vi "GTcode_v6_simulISS_MAP.vi"() -> ()   [LabVIEW 2016]
uses:
  <vilib>/Utility/error.llb/DialogType.ctl
  <vilib>/Analysis/5stat.llb/RMS (DBL).vi
  <vilib>/Utility/config.llb/Write Key (String).vi
  <vilib>/Utility/config.llb/Write Key (U32).vi
  <vilib>/Utility/config.llb/Write Key (Double).vi
  <vilib>/Utility/config.llb/Write Key (I32).vi
  <vilib>/Utility/config.llb/Read Key (U32).vi
  <vilib>/Utility/config.llb/Read Key (I32).vi
  <vilib>/Waveform/WDTOps.llb/WDT Append Waveforms DBL.vi
  <vilib>/Utility/file.llb/Write Delimited Spreadsheet (string).vi
  <vilib>/Waveform/WDTFileIO.llb/Export Waveforms To Spreadsheet File (1D).vi
  <vilib>/Utility/config.llb/NI_LVConfig.lvlib
  <vilib>/Analysis/NI_AALPro.lvlib
panel:
  out "MARk Wvfm":waveform(dbl)(graph)
  out "ComboMaxArray":dbl[](array[numeric])
  out "Trial Data Column Headers":string[](array[string])
  in  "TrialDataRowHeaders":string[](array[string])=["Wfm1", "Wfm2", "Wfm3", "Wfm4", "Wfm5", "Wfm6", "Wfm7", "Wfm8"]
  out "SignalMaxArray":dbl[][](array[numeric])
  in  "CurrentMaxIndex":dbl
  out "SignalsAvgMaxArray":dbl[](array[numeric])
  in  "Mean%Index":dbl=4.0
  in  "%StdDevIndex":dbl=5.0
  in  "StdDevIndex":dbl=3.0
  in  "MeanIndex":dbl=2.0
  in  "MaxIndex":dbl=1.0
  in  "MinIndex":dbl
  out "Stability Data":dbl[][](array[numeric])
  out "trialFilteredData":waveform(dbl)[](array[waveform])
  out "filteredWaveforms":waveform(dbl)[](array[waveform])
  in  "ComboMaxAvg":dbl
  in  "End Program":bool
  out "Wfm1":waveform(dbl)(graph)
  out "Wfm2":waveform(dbl)(graph)
  out "Wfm3":waveform(dbl)(graph)
  out "Wfm4":waveform(dbl)(graph)
  out "Wfm5":waveform(dbl)(graph)
  out "Wfm6":waveform(dbl)(graph)
  out "Wfm7":waveform(dbl)(graph)
  out "Wfm8":waveform(dbl)(graph)
  out "RMS 1":dbl(graph)
  out "RMS 2":dbl(graph)
  out "RMS 3":dbl(graph)
  out "RMS 4":dbl(graph)
  out "RMS 5":dbl(graph)
  out "RMS 6":dbl(graph)
  out "RMS 7":dbl(graph)
  out "RMS 8":dbl(graph)
  out "CombinedMovingAvg":dbl
  out "LeftPercentActivation":dbl
  out "GetMaxStartTime":timestamp
  out "Aggregate1":waveform(dbl)[](array[waveform])
  out "Aggregate2":waveform(dbl)[](array[waveform])
  out "Aggregate3":waveform(dbl)[](array[waveform])
  out "Aggregate4":waveform(dbl)[](array[waveform])
  out "Aggregate5":waveform(dbl)[](array[waveform])
  out "Aggregate6":waveform(dbl)[](array[waveform])
  out "Aggregate7":waveform(dbl)[](array[waveform])
  out "Aggregate 8":waveform(dbl)[](array[waveform])
  in  "Tab Control":T1(tab)=enum."Real Time Fitting Parameters"
  in  "Fixed Time":bool
  in  "Detector Used":T2(ring)=enum."Det 2"
  in  "Real Time Fitting?":bool
  out "g2":cluster{"Delay Time":sgl[], sgl[]}[](graph) caption="Normalized Correlation Function"
  out "Tau":cluster{"tmp":dbl, dbl}(graph) caption="Relative Changes of Flow"
  in  "QUIT":bool
  in  "Clear plots":bool
  in  "Baseline":bool
  in  "MARK\nMark":bool
  in  "Stop":bool
  in  "Sequence Scan":bool
  out "Mark #":u32
  out "Trial #":u32
  out "Frame #":u32
  out "Det 8":sgl format="%.3f"
  out "Det 7":sgl format="%.3f"
  out "Det 6":sgl format="%.3f"
  out "Det 5":sgl format="%.3f"
  out "Det 4":sgl format="%.3f"
  out "Det 3":sgl format="%.3f"
  out "Det 2":sgl format="%.3f"
  out "Det 1":sgl format="%.3f"
  out "Computer Time":string="2010-1-12 23:16:10"
  in  "D1":bool
  in  "D2":bool
  in  "D3":bool
  in  "D4":bool
  in  "D5":bool
  in  "D6":bool
  in  "D7":bool
  in  "D8":bool
  in  "Fixed # of Frames":u32=5
  out "Status":string="Quit"
  in  "Optical Switch OPEN":bool
  in  "Delay between frames(ms)":u32=500
  out "Time Left (ms)":sgl format="%.3f"
  in  "Integration Time (ms)":sgl=1000.0 min=1 max=13000 step=1
  in  "File Name:":string="test0"
  in  "Data Save Directory:":path=path "C:/data"
  in  "ISS Lasers ON":bool
  in  "Test":bool
  out "DispLeftMovingAvg":dbl(slide) caption="EMG" max=1.0 scale=0.0..100.0
  in  "startGetMax":bool
  in  "resetMax":bool
  out "Trial In Progress":bool
  out "Acquiring Max":bool
  in  "Lines":tag="Dev1/port1/line0:1, Dev1/port1/line3:7"
  in  "Delaytime(ms)":u32=200
  in  "Initialize Correlator":bool
  in  "Detector Select":enum32{"4 Detectors", "8 Detectors"}(radio)=enum."8 Detectors"
  in  "Update Time (ms)\nDO NOT CHANGE!":u32=105 min=1 max=999 step=1
  in  "Laser Input Name":refnum<visa-resource-name>="COM7"
  in  "Visible Averages":bool[](array[boolean])=[FALSE, FALSE, FALSE, FALSE]
  in  "Avg":bool[][](array[boolean])=[[FALSE, FALSE, FALSE, FALSE, FALSE, FALSE, FALSE, FALSE], [FALSE, FALSE, FALSE, FALSE, FALSE, FALSE, FALSE, FALSE], [FALSE, FALSE, FALSE, FALSE, FALSE, FALSE, FALSE, FALSE], [FALSE, FALSE, FALSE, FALSE, FALSE, FALSE, FALSE, FALSE]]
  in  "Number Samples":dbl=50.0
  out "NIBP Data (*scaled by 98 to convert from V to mmHg)":dynamicdata(graph)
  in  "Record MAP data?":bool=TRUE
  in  "Sampling Rate (Hz)":dbl=100.0
  in  "ExternalADC":tag="Dev2"
  in  "Lower Cut-Off":dbl=20.0
  in  "Upper Cut-Off":dbl=300.0
  in  "Sample rate (Hz)":dbl=2000.0
  in  "Frames Per Second":dbl=30.0
  in  "Moving Average Length (s)":dbl=0.5
  in  "SignalB":dbl=2.0
  in  "SignalA":dbl=1.0
  in  "Target Percentage":dbl=10.0
  in  "Amplitude Error":dbl
  in  "NumberOfMaximumsInAverage":dbl=3.0
  in  "SecondsToAcquireMax":dbl=10.0
  in  "EMG Input Device\nProduct Type":string="USB-6009"
  out "raw data":dynamicdata(graph)
  out "Combined RMS":dbl(graph)
  out "Trial Raw Waveforms":waveform(dbl)[](graph)
  out "Bufffer Index":dbl
  out "Frames in Buffer":dbl
  out "Samples per frame":dbl
  out "Reset Data Acquisition\nAnd UI Updating":bool=TRUE
  in  "Extension":string="_EMG.txt"
  out "4CH?":bool
  out "Detector#":u32=1
  out "Source#":u32=1
  # "kHz"
  # "kHz"
  # "Maximums Data"
  # "Don't Change these Parameters unless you know clearly what you are doing"
  # "ISS Triggers Setup"
  # "Channel Parameters"
  # "Step1"
  # "Line"
  # "0"
  # "1"
  # "3"
  # "4"
  # "5"
  # "6"
  # "7"
  # "*The number of lines in the list must\nmatch the number of elements in\nthe array."
  # "Step2"
  # "Line"
  # "0"
  # "1"
  # "3"
  # "4"
  # "5"
  # "6"
  # "7"
  # "Step3"
  # "Line"
  # "0"
  # "1"
  # "3"
  # "4"
  # "5"
  # "6"
  # "7"
  # "Line    Signal\n\n0           ISS Trigger (0: OFF, 1: ON)\n1           Flow Laser 1 ON/OFF (0:OFF, 1:ON)\n2           ISS Data Acquisition (0: DONE, 1: NO)\n3           ISS Laser ON/OFF (0: ON, 1: OFF)\n4           Trigger for Marks  (0: OFF, 1: ON)\n5           Flow Laser 2 ON/OFF (0:OFF, 1:ON)\n6           Reserved\n7           Reserved"
  # "Wait ISS Data Acuisition DONE Signal"
  # "Step4"
  # "Step5"
  # "Line"
  # "0"
  # "1"
  # "3"
  # "4"
  # "5"
  # "6"
  # "7"
  # "Flow Lasers Setup"
  # "FROM FRONT PANEL"
  # "Line"
  # "0"
  # "1"
  # "3"
  # "4"
  # "5"
  # "6"
  # "7"
  # "Line"
  # "0"
  # "1"
  # "3"
  # "4"
  # "5"
  # "6"
  # "7"
  # "Det 1"
  # "Det 2"
  # "Det 3"
  # "Det 4"
  # "Det 5"
  # "Det 6"
  # "Det 7"
  # "Det 8"
  # "Avg 1"
  # "Avg 2"
  # "Avg 3"
  # "Avg 4"
  # "Db"
  # "Beta"
  # "Mua"
  # "MuS'"
  # "1"
  # "2"
  # "3"
  # "4"
  # "5"
  # "6"
  # "7"
  # "8"
  # "Avg 1"
  # "Starting Pt"
  # "End Pt"
  # "Approximate"
  # "Variables"
  # "Avg 2"
  # "Avg 3"
  # "Avg 4"
  # "Source Detector  Separations"
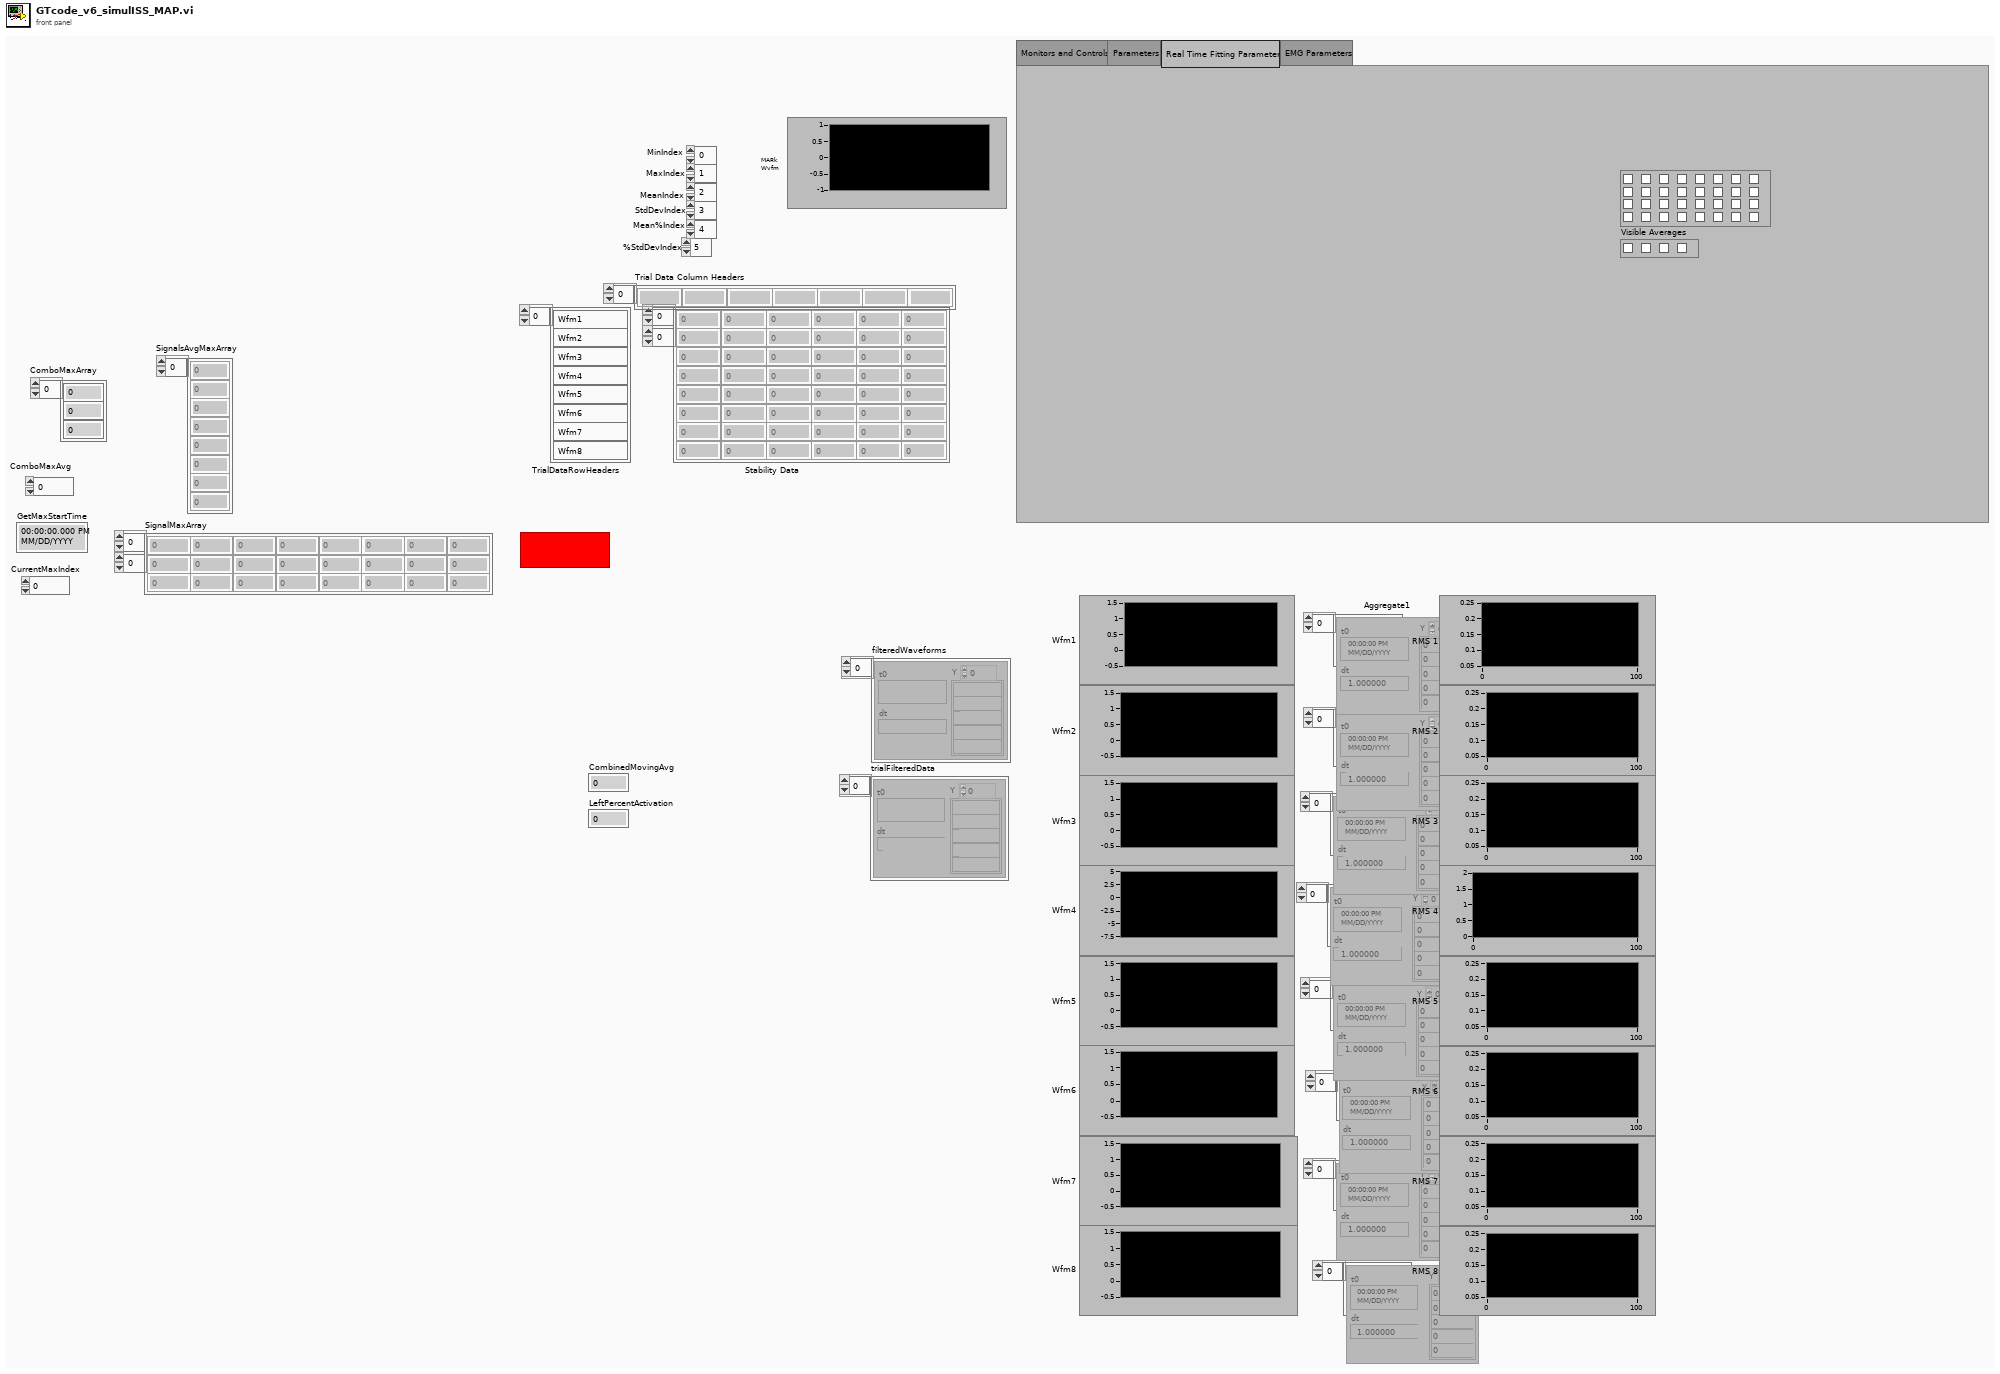
[diagram p1: front panel]
types:
  T1 = enum32{"Monitors and Controls", "Parameters", "Real Time Fitting Parameters", "EMG Parameters"}
  T2 = enum16{"Det 1", "Det 2", "Det 3", "Det 4", "Det 5", "Det 6", "Det 7", "Det 8"}
  T3 = typedef "DialogType.ctl" = u16
  T4 = typedef "WaveformArrayControl.ctl" = waveform(dbl)[]
  T5 = enum8{"Enabled", "Disabled", "Disabled and Grayed Out"}
  T6 = cluster{dbl, dbl, dbl, dbl, dbl, dbl, dbl, dbl, dbl, dbl, dbl, dbl}
  T7 = typedef "NI_LVConfig.lvlib/Config Data RefNum.ctl" = refnum<k1>
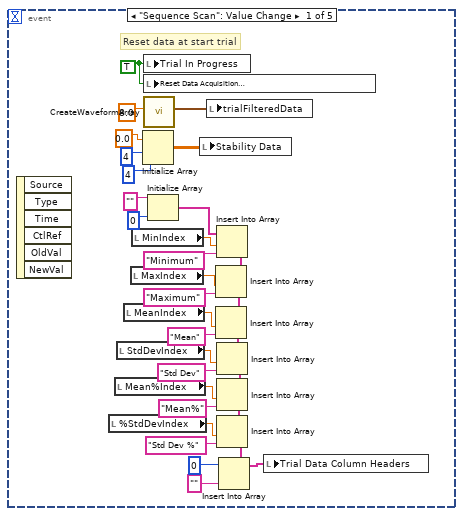
[diagram p2: hidden frame]
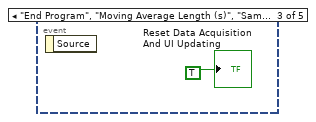
[diagram p5: hidden frame]
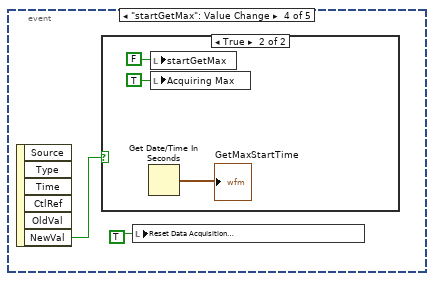
[diagram p6: hidden frame]
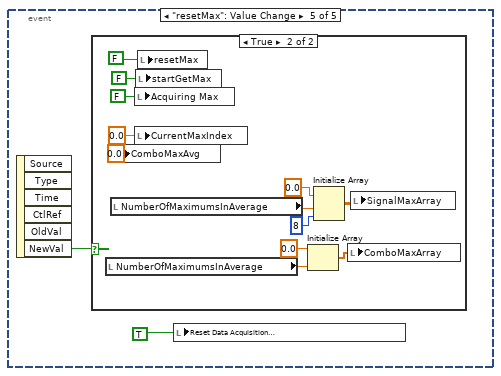
[diagram p8: hidden frame]
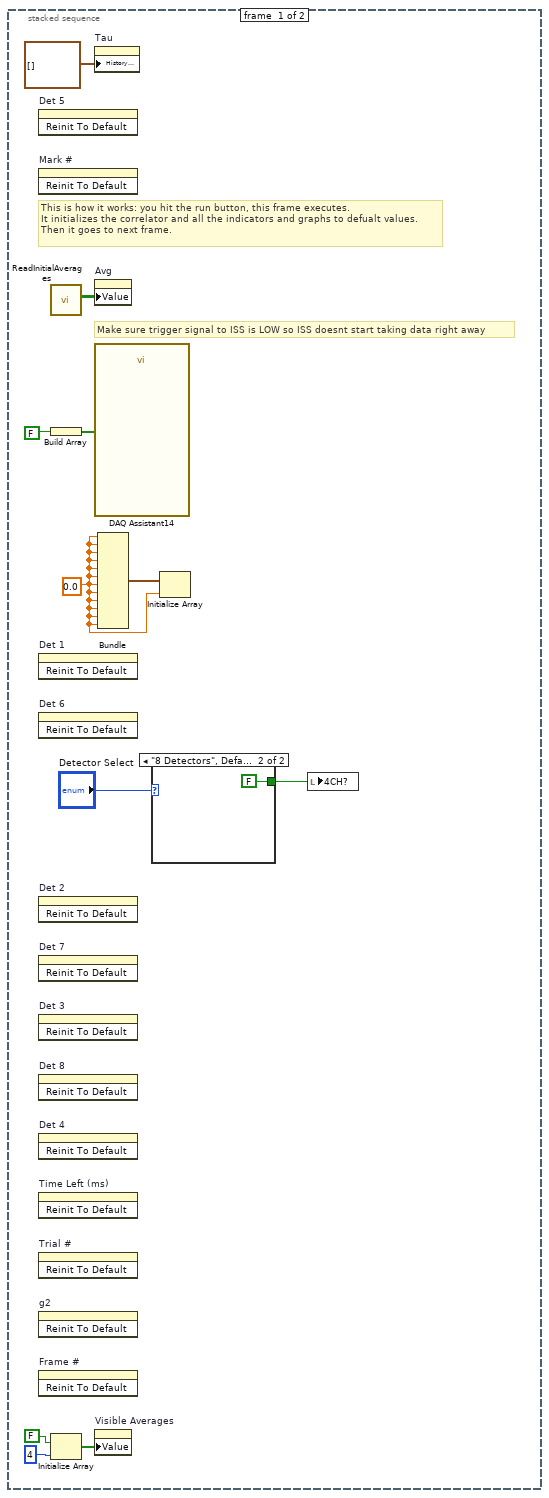
[diagram p15: hidden frame]
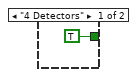
[diagram p16: hidden frame]
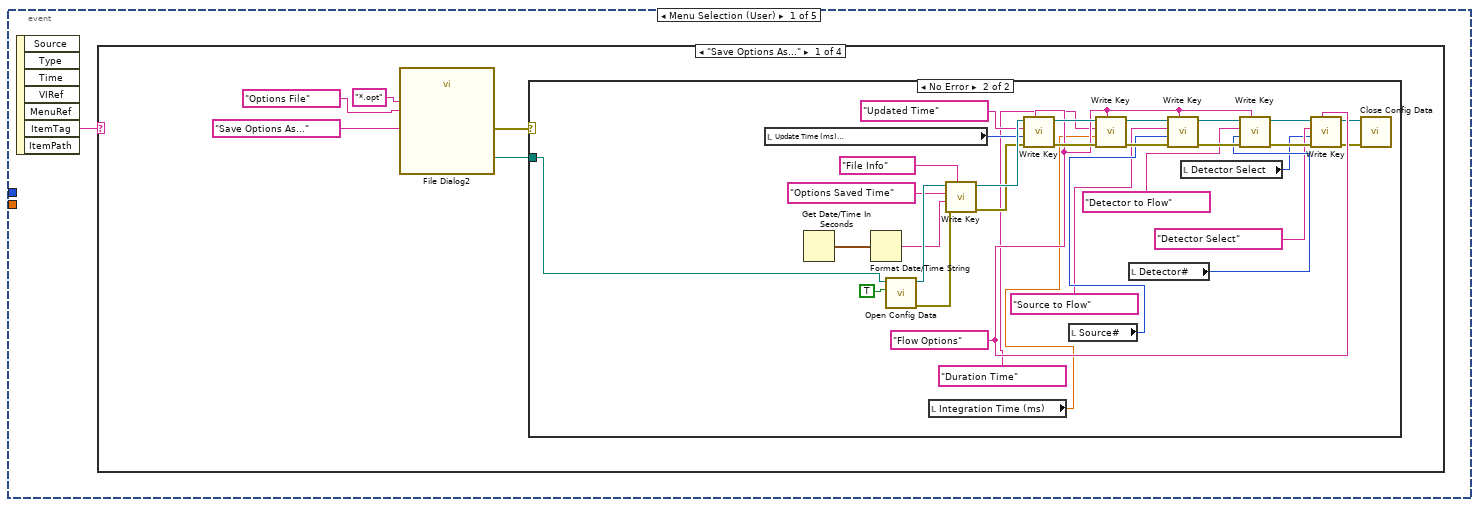
[diagram p17: hidden frame]
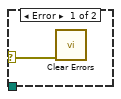
[diagram p18: hidden frame]
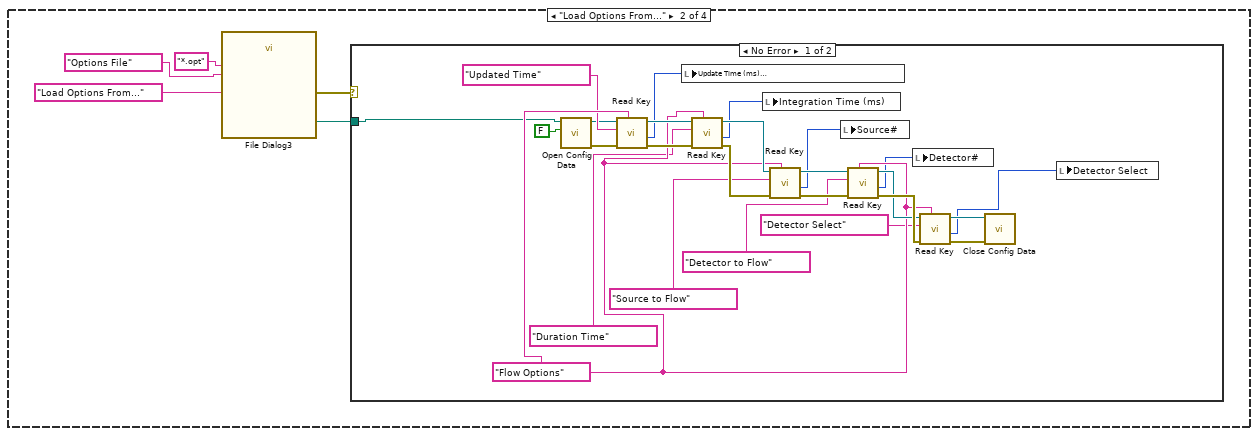
[diagram p19: hidden frame]
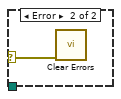
[diagram p20: hidden frame]
diagram:
  # "Calculate Stability of data"
  # "Acquire MAX"
  # "Filtering and updating variables"
  # "Saving Trial Data"
  n1 = local read "NumberOfMaximumsInAverage"() -> (w5:dbl)
  n2 = local read "NumberOfMaximumsInAverage"() -> (w1:dbl)
  n3 = Initialize Array(0.0 ("element"), w5, 8 ("dimension size")) -> (→"SignalMaxArray":dbl[][])
  n4 = Initialize Array(0.0 ("element"), w1) -> (→"ComboMaxArray":dbl[])
  n5 = while {
    stop <- "End Program" stop-if-true
    # "Grab Relevant Sample from Moving Average, Update UI, Save Data if necessary"
    # "Initialize Buffers"
    # "Listen for settings changes and restart runtime loop\nAlso make updates for trial changes"
    n6 = local read "Frames Per Second"() -> (w19:dbl)
    n7 = local read "Frames Per Second"() -> (w22:dbl)
    n8 = local read "Moving Average Length (s)"() -> (w20:dbl)
    n9 = local read "Sample rate (Hz)"() -> (w23:dbl)
    n10 = local write "Reset Data Acquisition\nAnd UI Updating"(FALSE) -> ()
    n11 = Divide(x=w23, y=w22) -> (x/y=→"Samples per frame":dbl)
    n12 = Multiply(x=w20, y=w19) -> (x*y=w16:dbl)
    "Frames in Buffer" <- w16
    n13 = call "GetDevice.vi"("EMG Input Device\nProduct Type"="EMG Input Device\nProduct Type") -> ("DAQmx Device Name"=w12:tag)  [unwired: 10 in]
    n14 = while {
      tunnel: w12 -> [w172]
      stop <- w218 stop-if-true
      n15 = local read "Reset Data Acquisition\nAnd UI Updating"() -> (w218:bool)
      n16 = local read "Trial In Progress"() -> (w176:bool)
      n17 = case shown="True" w176 {
        frame False {
        }
        frame True {
          # "Start aggregating data for trial"
          n18 = local read "SignalsAvgMaxArray"() -> (w251:dbl[])
          n19 = local read "MeanIndex"() -> (w255:dbl)
          n20 = local read "trialFilteredData"() -> (w258:waveform(dbl)[])
          n21 = local read "filteredWaveforms"() -> (w259:waveform(dbl)[])
          n22 = local read "MinIndex"() -> (w257:dbl)
          n23 = local read "MaxIndex"() -> (w256:dbl)
          n24 = local read "StdDevIndex"() -> (w254:dbl)
          n25 = local read "Mean%Index"() -> (w253:dbl)
          n26 = local read "%StdDevIndex"() -> (w252:dbl)
          n27 = for {
            tunnel: w259 -> [w269] mode=indexing
            tunnel: w258 -> [w270] mode=indexing
            tunnel: [w268] -> w249 mode=indexing
            tunnel: [w260] -> w250 mode=indexing
            tunnel: w257 -> [w267]
            tunnel: w256 -> [w266]
            tunnel: w255 -> [w265]
            tunnel: w254 -> [w264]
            tunnel: w253 -> [w263]
            tunnel: w252 -> [w262]
            tunnel: w251 -> [w261] mode=indexing
            n28 = call-poly <vilib>:"Append Waveforms.vi"("waveform B"=w269, "waveform A"=w270) -> ("waveform out"=w268:waveform(dbl))  [unwired: 8 in, 1 out]
            n29 = call "GetStabilityData.vi"("ProvidedData"=w268, "ScaleMax"=w261, "MinIndex"=w267, "MaxIndex"=w266, "MeanIndex"=w265, "StdDevIndex"=w264, "Mean%Index"=w263, "%StdDevIndex"=w262) -> ("ReturnData"=w260:dbl[])  [unwired: 7 in]
          }
          n30 = local write "trialFilteredData"(w249) -> ()
          n31 = local write "Stability Data"(w250) -> ()
        }
      }
      n32 = local read "Sample rate (Hz)"() -> (w225:dbl)
      n33 = local read "Samples per frame"() -> (w224:dbl)
      n34 = local read "Aggregate 8"() -> (w174:waveform(dbl)[])
      n35 = local read "Reset Data Acquisition\nAnd UI Updating"() -> (w217:bool)
      n36 = local read "raw data"() -> (w223:dynamicdata)
      n37 = local read "Bufffer Index"() -> (w199:dbl)
      n38 = local read "Frames in Buffer"() -> (w220:dbl)
      n39 = local read "Aggregate1"() -> (w198:waveform(dbl)[])
      n40 = local read "Aggregate2"() -> (w196:waveform(dbl)[])
      n41 = local read "Aggregate3"() -> (w194:waveform(dbl)[])
      n42 = local read "Aggregate4"() -> (w192:waveform(dbl)[])
      n43 = local read "Aggregate5"() -> (w190:waveform(dbl)[])
      n44 = local read "Aggregate6"() -> (w188:waveform(dbl)[])
      n45 = local read "Aggregate7"() -> (w186:waveform(dbl)[])
      n46 = local read "Acquiring Max"() -> (w169:bool)
      n47 = case shown="True" w169 {
        frame False {
        }
        frame True {
          # "Update\nMax\nIf \nAcquiring\nMax"
          n48 = local read "filteredWaveforms"() -> (w237:waveform(dbl)[])
          n49 = local read "SignalMaxArray"() -> (w236:dbl[][])
          n50 = local read "CurrentMaxIndex"() -> (w235:dbl)
          n51 = local read "GetMaxStartTime"() -> (w233:timestamp)
          n52 = local read "SecondsToAcquireMax"() -> (w230:dbl)
          n53 = Get Date/Time In Seconds() -> (seconds since 1Jan1904=w232:timestamp)
          n54 = Subtract(x=w232, y=w233) -> (x-y=w231:dbl)
          n55 = Index Array(array=w236, index (row)=w235) -> (element=w238:dbl[])  [unwired: 1 in]
          n56 = Less?(x=w231, y=w230) -> (x < y?=w226:bool)
          n57 = for {
            tunnel: w238 -> [w246] mode=indexing
            tunnel: w237 -> [w248] mode=indexing
            tunnel: [w245] -> w234 mode=indexing
            n58 = call "ArrayMax.vi"("Array"=w248) -> ("max"=w247:dbl)  [unwired: 10 in]
            n59 = call "MaxValue.vi"("NewValue"=w247, "CurrentMax"=w246) -> ("Max"=w245:dbl)  [unwired: 9 in]
          }
          n60 = case shown="False" w226 {
            frame False {
              n61 = local read "CurrentMaxIndex"() -> (w240:dbl)
              n62 = local read "NumberOfMaximumsInAverage"() -> (w242:dbl)
              n63 = Increment(x=w240) -> (x+1=w241:dbl)
              n64 = Quotient & Remainder(x=w241, y=w242) -> (x-y*floor(x/y)=w239:dbl)  [unwired: 1 out]
              n65 = local write "CurrentMaxIndex"(w239) -> ()
            }
            frame True {
            }
          }
          n66 = local write "Acquiring Max"(w226) -> ()
          n67 = Replace Array Subset(array=w236, new element=w234, index (row)=w235) -> (w229:dbl[][])  [unwired: 1 in]
          n68 = Transpose 2D Array(2D array=w229) -> (transposed array=w228:dbl[][])
          n69 = for {
            tunnel: w228 -> [w244] mode=indexing
            tunnel: [w243] -> w227 mode=indexing
            n70 = call "ArrayMean.vi"("Array"=w244) -> ("Mean"=w243:dbl)  [unwired: 10 in]
          }
          n71 = local write "SignalsAvgMaxArray"(w227) -> ()
          n72 = local write "SignalMaxArray"(w229) -> ()
        }
      }
      n73 = local read "Wfm1"() -> (w197:waveform(dbl))
      n74 = local read "Wfm2"() -> (w195:waveform(dbl))
      n75 = local read "Wfm3"() -> (w193:waveform(dbl))
      n76 = local read "Wfm4"() -> (w191:waveform(dbl))
      n77 = local read "Wfm5"() -> (w189:waveform(dbl))
      n78 = local read "Wfm6"() -> (w187:waveform(dbl))
      n79 = local read "Wfm7"() -> (w185:waveform(dbl))
      n80 = local read "Wfm8"() -> (w184:waveform(dbl))
      n81 = local read "Mark #"() -> (w164:u32)
      n82 = call "Filter"("Lower Cut-Off"="Lower Cut-Off", "Upper Cut-Off"="Upper Cut-Off", "Signal"=w223) -> ("Filtered Signal"=w166:dynamicdata)  [unwired: 7 in, 1 out]
      n83 = Merge Signals(w166, w164) -> (w165:dynamicdata)
      n84 = call "Convert from Dynamic Data9"("Dynamic Data Type"=w165) -> ("Array of Waveform"=w171:waveform(dbl)[])  [unwired: 3 in]
      n85 = Increment(x=w199) -> (x+1=w219:dbl)
      n86 = Replace Array Subset(array=w188, new element=w187, index=w199) -> (w178:waveform(dbl)[])
      n87 = Replace Array Subset(array=w186, new element=w185, index=w199) -> (w177:waveform(dbl)[])
      n88 = Replace Array Subset(array=w174, new element=w184, index=w199) -> (w175:waveform(dbl)[])
      n89 = Replace Array Subset(array=w190, new element=w189, index=w199) -> (w179:waveform(dbl)[])
      n90 = Replace Array Subset(array=w192, new element=w191, index=w199) -> (w180:waveform(dbl)[])
      n91 = Replace Array Subset(array=w198, new element=w197, index=w199) -> (w183:waveform(dbl)[])
      n92 = Replace Array Subset(array=w196, new element=w195, index=w199) -> (w182:waveform(dbl)[])
      n93 = Replace Array Subset(array=w194, new element=w193, index=w199) -> (w181:waveform(dbl)[])
      n94 = Split Signals(w165) -> (w215:dynamicdata, w214:dynamicdata, w213:dynamicdata, w212:dynamicdata, w211:dynamicdata, w210:dynamicdata, w209:dynamicdata, w208:dynamicdata, w167:dynamicdata)  [unwired: 9 in]
      n95 = call "Convert from Dynamic Data10"("Dynamic Data Type"=w167) -> ("Waveform"=→"MARk Wvfm":waveform(dbl))  [unwired: 3 in]
      n96 = Absolute Value(x=w171) -> (abs(x)=w170:waveform(dbl)[])
      n97 = call "DAQ Assistant16"("rate"=w225, "number of samples"=w224, "stop (T)"=w217, "device name"=w172) -> ("data"=→"raw data":dynamicdata)  [unwired: 13 in, 2 out]
      n98 = Quotient & Remainder(x=w219, y=w220) -> (x-y*floor(x/y)=w221:dbl)  [unwired: 1 out]
      n99 = local write "filteredWaveforms"(w170) -> ()
      n100 = local write "Aggregate 8"(w175) -> ()
      n101 = local write "Bufffer Index"(w221) -> ()
      n102 = local write "Aggregate6"(w178) -> ()
      n103 = local write "Aggregate3"(w181) -> ()
      n104 = local write "Aggregate7"(w177) -> ()
      n105 = local write "Aggregate4"(w180) -> ()
      n106 = local write "Aggregate5"(w179) -> ()
      n107 = local write "Aggregate1"(w183) -> ()
      n108 = local write "Aggregate2"(w182) -> ()
      n109 = call "Convert from Dynamic Data"("Dynamic Data Type"=w215) -> ("Waveform"=→"Wfm1":waveform(dbl))  [unwired: 3 in]
      n110 = call "Convert from Dynamic Data2"("Dynamic Data Type"=w214) -> ("Waveform"=→"Wfm2":waveform(dbl))  [unwired: 3 in]
      n111 = call "Convert from Dynamic Data3"("Dynamic Data Type"=w213) -> ("Waveform"=→"Wfm3":waveform(dbl))  [unwired: 3 in]
      n112 = call "Convert from Dynamic Data8"("Dynamic Data Type"=w212) -> ("Waveform"=→"Wfm4":waveform(dbl))  [unwired: 3 in]
      n113 = call "Convert from Dynamic Data4"("Dynamic Data Type"=w211) -> ("Waveform"=→"Wfm5":waveform(dbl))  [unwired: 3 in]
      n114 = call "Convert from Dynamic Data5"("Dynamic Data Type"=w210) -> ("Waveform"=→"Wfm6":waveform(dbl))  [unwired: 3 in]
      n115 = call "Convert from Dynamic Data6"("Dynamic Data Type"=w209) -> ("Waveform"=→"Wfm7":waveform(dbl))  [unwired: 3 in]
      n116 = call "Convert from Dynamic Data7"("Dynamic Data Type"=w208) -> ("Waveform"=→"Wfm8":waveform(dbl))  [unwired: 3 in]
    }
    n117 = call "CreateWaveformArray.vi"("bufferSize"=w16) -> ("initialized array"=→"Aggregate1" →"Aggregate2" →"Aggregate3" →"Aggregate4" →"Aggregate5" →"Aggregate6" →"Aggregate7" →"Aggregate 8":waveform(dbl)[])  [unwired: 5 in, 1 out]
    n118 = event shown="[1] \"Stop\": Value Change" {
      selector: _ -> [_ _ _ _ _]
      dyn-events: _ -> [_ _ _ _ _]
      timeout: _ -> [_ _ _ _ _]
      event "Sequence Scan": Value Change {
        w54 = TRUE ("Trial In Progress")
        # "Reset data at start trial"
        n119 = event-data() -> ()  [unwired: 1 in, 6 out]
        n120 = local read "%StdDevIndex"() -> (w30:dbl)
        n121 = local read "Mean%Index"() -> (w31:dbl)
        n122 = local read "StdDevIndex"() -> (w35:dbl)
        n123 = local read "MeanIndex"() -> (w39:dbl)
        n124 = local read "MaxIndex"() -> (w42:dbl)
        n125 = local read "MinIndex"() -> (w44:dbl)
        n126 = Initialize Array(0.0 ("element"), 4 ("dimension size"), 4 ("dimension size")) -> (w48:dbl[][])
        n127 = local write "Trial In Progress"(w54) -> ()
        n128 = local write "Reset Data Acquisition\nAnd UI Updating"(w54) -> ()
        n129 = call "CreateWaveformArray.vi"("bufferSize"=8.0) -> ("initialized array"=w53:waveform(dbl)[])  [unwired: 5 in, 1 out]
        n130 = Initialize Array("", 0 ("dimension size")) -> (w43:string[])
        n131 = local write "Stability Data"(w48) -> ()
        n132 = local write "trialFilteredData"(w53) -> ()
        n133 = Insert Into Array(array=w43, index=w44, new element="Minimum" ("new element/subarray")) -> (w40:string[])
        n134 = Insert Into Array(array=w40, index=w42, new element="Maximum" ("new element/subarray")) -> (w37:string[])
        n135 = Insert Into Array(array=w37, index=w39, new element="Mean" ("new element/subarray")) -> (w34:string[])
        n136 = Insert Into Array(array=w34, index=w35, new element="Std Dev" ("new element/subarray")) -> (w32:string[])
        n137 = Insert Into Array(array=w32, index=w31, new element="Mean%" ("new element/subarray")) -> (w28:string[])
        n138 = Insert Into Array(array=w28, index=w30, new element="Std Dev %" ("new element/subarray")) -> (w25:string[])
        n139 = Insert Into Array(array=w25, index=0, new element="" ("new element/subarray")) -> (w26:string[])
        n140 = local write "Trial Data Column Headers"(w26) -> ()
      }
      event "Stop": Value Change {
        # "Only Execute if Trial Already in progress"
        n141 = event-data() -> ()  [unwired: 1 in, 6 out]
        n142 = local read "Trial In Progress"() -> (w56:bool)
        n143 = case shown="True" w56 {
          frame False {
          }
          frame True {
            w75 = T3 2 items=["no dialog", "OK message", "continue or stop message", "OK message + warnings", "continue/stop + warnings"] ("type of dialog (OK msg:1)")
            (unwired) 1 items=["no exception", "cancel error on match", "set error on match"] ("[exception action] (none:0)")
            (unwired) 1430 ("[exception code]")
            # "Append Waveform Data"
            # "Write Stability Data"
            # "End Trial and save data, create directory if needed"
            n144 = local read "Data Save Directory:"() -> (w76:path)
            n145 = local read "Trial Data Column Headers"() -> (w63:string[])
            n146 = local read "File Name:"() -> (w72:string)
            n147 = local read "Stability Data"() -> (w59:dbl[][])
            n148 = local read "Extension"() -> (w73:string)
            n149 = local read "TrialDataRowHeaders"() -> (w62:string[])
            n150 = local read "trialFilteredData"() -> (w65:waveform(dbl)[])
            n151 = local write "Trial In Progress"(FALSE ("Trial In Progress")) -> ()
            n152 = for {
              tunnel: w59 -> [w81] mode=indexing
              tunnel: [w80] -> w57 mode=indexing
              n153 = for {
                tunnel: w81 -> [w83] mode=indexing
                tunnel: [w82] -> w80 mode=indexing
                n154 = Format Into String(format string="%f", w83) -> (resulting string=w82:string)  [unwired: 2 in, 1 out]
              }
            }
            n155 = call <vilib>:"Check if File or Folder Exists.vi"("path"=w76) -> ("file or folder exists?"=w78:bool, "dup path"=w77:path)  [unwired: 8 in, 1 out]
            n156 = case shown="False" w78 {
              tunnel: [w85 w87] -> w74
              tunnel: w77 -> [w86 w87]
              frame False {
                n157 = Create Folder(path (use dialog)=w86) -> (created path=w85:path)  [unwired: 2 in, 2 out]
              }
              frame True {
              }
            }
            n158 = Concatenate Strings(w72, w73) -> (w71:string)
            n159 = Build Path(base path=w74, name or relative path=w71) -> (appended path=w68:path)
            n160 = Insert Into Array(array=w57, index (col)=0 ("index (row)"), new element=w62) -> (w69:string[][])  [unwired: 1 in]
            n161 = Insert Into Array(array=w69, index (row)=0 ("index (col)"), new element=w63) -> (w58:string[][])  [unwired: 1 in]
            n162 = call-poly <vilib>:"Write Delimited Spreadsheet.vi"("file path (dialog if empty)"=w68, "2D data"=w58, "append to file? (new file:F)"=FALSE) -> ("new file path (Not A Path if cancelled)"=w66:path)  [unwired: 11 in, 1 out]
            n163 = call-poly <vilib>:"Export Waveforms to Spreadsheet File.vi"("append to file? (new file:F)"=TRUE, "waveforms"=w65, "file path (dialog if empty)"=w66) -> ("error out"=w70:errorcluster)  [unwired: 7 in, 1 out]
            n164 = call <vilib>:"General Error Handler.vi"("type of dialog (OK msg:1)"=w75, "error in (no error)"=w70) -> ()  [unwired: 9 in, 5 out]
          }
        }
        n165 = local write "Reset Data Acquisition\nAnd UI Updating"(TRUE ("Reset Data Acquisition\nAnd UI Updating")) -> ()
      }
      event "End Program", "Moving Average Length (s)", "Sample rate (Hz)", "Frames Per Second": Value Change {
        n166 = event-data() -> ()  [unwired: 1 in, 1 out]
        "Reset Data Acquisition\nAnd UI Updating" <- TRUE
      }
      event "startGetMax": Value Change {
        n167 = event-data() -> ("NewVal"=w90:bool)  [unwired: 1 in, 5 out]
        n168 = case shown="True" w90 {
          frame False {
          }
          frame True {
            n169 = Get Date/Time In Seconds() -> (seconds since 1Jan1904=→"GetMaxStartTime":timestamp)
            n170 = local write "startGetMax"(FALSE) -> ()
            n171 = local write "Acquiring Max"(TRUE ("Acquiring Max")) -> ()
          }
        }
        n172 = local write "Reset Data Acquisition\nAnd UI Updating"(TRUE ("Reset Data Acquisition\nAnd UI Updating")) -> ()
      }
      event "resetMax": Value Change {
        n173 = event-data() -> ("NewVal"=w95:bool)  [unwired: 1 in, 5 out]
        n174 = case shown="True" w95 {
          frame False {
          }
          frame True {
            n175 = local read "NumberOfMaximumsInAverage"() -> (w98:dbl)
            n176 = local read "NumberOfMaximumsInAverage"() -> (w101:dbl)
            n177 = local write "ComboMaxAvg"(0.0 ("Left Max")) -> ()
            n178 = local write "Acquiring Max"(FALSE ("Acquiring Max")) -> ()
            n179 = local write "CurrentMaxIndex"(0.0 ("CurrentMaxIndex")) -> ()
            n180 = local write "startGetMax"(FALSE ("startGetMax")) -> ()
            n181 = local write "resetMax"(FALSE ("endGetMax")) -> ()
            n182 = Initialize Array(0.0 ("element"), w98) -> (w97:dbl[])
            n183 = Initialize Array(0.0 ("element"), w101, 8 ("dimension size")) -> (w102:dbl[][])
            n184 = local write "ComboMaxArray"(w97) -> ()
            n185 = local write "SignalMaxArray"(w102) -> ()
          }
        }
        n186 = local write "Reset Data Acquisition\nAnd UI Updating"(TRUE ("Reset Data Acquisition\nAnd UI Updating")) -> ()
      }
    }
    n187 = while {
      stop <- w153 stop-if-true
      # "Update Displays -> Left and Right percent activbation as well as 2D activation graph Point Position"
      # "Get Moving Average Sample"
      # "Rectify"
      n188 = local read "Bufffer Index"() -> (w150:dbl)
      n189 = local read "Frames in Buffer"() -> (w149:dbl)
      n190 = local read "Acquiring Max"() -> (w108:bool)
      n191 = case shown="True" w108 {
        frame False {
        }
        frame True {
          n192 = local read "ComboMaxArray"() -> (w158:dbl[])
          n193 = local read "CurrentMaxIndex"() -> (w157:dbl)
          n194 = local read "CombinedMovingAvg"() -> (w154:dbl)
          n195 = Index Array(array=w158, index=w157) -> (element=w156:dbl)
          n196 = Greater?(x=w154, y=w156) -> (0:w155:bool)
          n197 = case shown="True" w155 {
            tunnel: w154 -> [_ w161]
            frame False {
            }
            frame True {
              n198 = local read "CurrentMaxIndex"() -> (w162:dbl)
              n199 = local read "ComboMaxArray"() -> (w163:dbl[])
              n200 = Replace Array Subset(array=w163, new element=w161, index=w162) -> (w159:dbl[])
              n201 = local write "ComboMaxArray"(w159) -> ()
              n202 = call "ArrayMean.vi"("Array"=w159) -> ("Mean"=w160:dbl)  [unwired: 10 in]
              n203 = local write "ComboMaxAvg"(w160) -> ()
            }
          }
        }
      }
      n204 = local read "Aggregate1"() -> (w148:waveform(dbl)[])
      n205 = local read "Aggregate2"() -> (w144:waveform(dbl)[])
      n206 = local read "Aggregate3"() -> (w147:waveform(dbl)[])
      n207 = local read "Aggregate4"() -> (w143:waveform(dbl)[])
      n208 = local read "Aggregate5"() -> (w146:waveform(dbl)[])
      n209 = local read "Aggregate6"() -> (w145:waveform(dbl)[])
      n210 = local read "Aggregate7"() -> (w142:waveform(dbl)[])
      n211 = local read "Aggregate 8"() -> (w141:waveform(dbl)[])
      n212 = local read "CombinedMovingAvg"() -> (w121:dbl)
      n213 = local read "trialFilteredData"() -> (→"Trial Raw Waveforms":waveform(dbl)[])
      n214 = local read "Frames Per Second"() -> (w152:dbl)
      n215 = local read "ComboMaxAvg"() -> (w120:dbl)
      n216 = local read "Reset Data Acquisition\nAnd UI Updating"() -> (w153:bool)
      n217 = call "GetSubarrayOfCircularBuffer.vi"("initialized array"=w142, "buffer size"=w149, "subset size"=w149, "start index"=w150) -> ("initialized array 2"=w110:T4)  [unwired: 7 in]
      n218 = call "GetSubarrayOfCircularBuffer.vi"("initialized array"=w141, "buffer size"=w149, "subset size"=w149, "start index"=w150) -> ("initialized array 2"=w109:T4)  [unwired: 7 in]
      n219 = call "GetSubarrayOfCircularBuffer.vi"("initialized array"=w147, "buffer size"=w149, "subset size"=w149, "start index"=w150) -> ("initialized array 2"=w114:T4)  [unwired: 7 in]
      n220 = call "GetSubarrayOfCircularBuffer.vi"("initialized array"=w143, "buffer size"=w149, "subset size"=w149, "start index"=w150) -> ("initialized array 2"=w113:T4)  [unwired: 7 in]
      n221 = call "GetSubarrayOfCircularBuffer.vi"("initialized array"=w146, "buffer size"=w149, "subset size"=w149, "start index"=w150) -> ("initialized array 2"=w112:T4)  [unwired: 7 in]
      n222 = call "GetSubarrayOfCircularBuffer.vi"("initialized array"=w145, "buffer size"=w149, "subset size"=w149, "start index"=w150) -> ("initialized array 2"=w111:T4)  [unwired: 7 in]
      n223 = Divide(x=w121, y=w120) -> (x/y=w122:dbl)
      n224 = call "GetSubarrayOfCircularBuffer.vi"("initialized array"=w148, "buffer size"=w149, "subset size"=w149, "start index"=w150) -> ("initialized array 2"=w116:T4)  [unwired: 7 in]
      n225 = call "GetSubarrayOfCircularBuffer.vi"("initialized array"=w144, "buffer size"=w149, "subset size"=w149, "start index"=w150) -> ("initialized array 2"=w115:T4)  [unwired: 7 in]
      n226 = Multiply(x=w122, y=100) -> (x*y=→"DispLeftMovingAvg" →"LeftPercentActivation":dbl)
      n227 = call-poly <vilib>:"RMS.vi"("X"=w116) -> ("rms value"=w135:dbl)  [unwired: 1 out]
      "RMS 1" <- w135
      n228 = call-poly <vilib>:"RMS.vi"("X"=w114) -> ("rms value"=w140:dbl)  [unwired: 1 out]
      "RMS 3" <- w140
      n229 = call-poly <vilib>:"RMS.vi"("X"=w113) -> ("rms value"=w139:dbl)  [unwired: 1 out]
      "RMS 4" <- w139
      n230 = call-poly <vilib>:"RMS.vi"("X"=w112) -> ("rms value"=w138:dbl)  [unwired: 1 out]
      "RMS 5" <- w138
      n231 = call-poly <vilib>:"RMS.vi"("X"=w111) -> ("rms value"=w137:dbl)  [unwired: 1 out]
      "RMS 6" <- w137
      n232 = call-poly <vilib>:"RMS.vi"("X"=w110) -> ("rms value"=w136:dbl)  [unwired: 1 out]
      "RMS 7" <- w136
      n233 = call-poly <vilib>:"RMS.vi"("X"=w109) -> ("rms value"=w133:dbl)  [unwired: 1 out]
      "RMS 8" <- w133
      n234 = call-poly <vilib>:"RMS.vi"("X"=w115) -> ("rms value"=w134:dbl)  [unwired: 1 out]
      "RMS 2" <- w134
      n235 = call "FramesPerSecondTOMilliseconds.vi"("Thermometer\nFps"=w152) -> ("x*y"=w117:dbl)  [unwired: 10 in]
      n236 = Wait (ms)(milliseconds to wait=w117) -> ()  [unwired: 1 out]
      n237 = Build Array(w135, w134, w140, w139, w138, w137, w136, w133) -> (w132:dbl[])
      n238 = Decrement(x="SignalA") -> (x-1=w124:dbl)
      n239 = Decrement(x="SignalB") -> (x-1=w126:dbl)
      n240 = Index Array(array=w132, index=w124) -> (element=w131:dbl)
      n241 = Index Array(array=w132, index=w126) -> (element=w130:dbl)
      n242 = Add(x=w131, y=w130) -> (x+y=w129:dbl)
      n243 = Divide(x=w129, y=2.0) -> (x/y=→"Combined RMS" →"CombinedMovingAvg":dbl)
    }
    n244 = local write "Reset Data Acquisition\nAnd UI Updating"("End Program") -> ()
    "Bufffer Index" <- 0.0 ("Bufffer Index")
  }
  n245 = stacked-sequence {
    frame #0 {
      w275 = 0.0
      # "Make sure trigger signal to ISS is LOW so ISS doesnt start taking data right away"
      # "This is how it works: you hit the run button, this frame executes.\nIt initializes the correlator and all the indicators and graphs to defualt values.\nThen it goes to next frame."
      n246 = invoke on="Det 5" class="DigNum (strict)" method="Reinit To Default"() -> ()  [unwired: 3 in, 3 out]
      n247 = invoke on="Mark #" class="DigNum (strict)" method="Reinit To Default"() -> ()  [unwired: 3 in, 3 out]
      n248 = invoke on="Det 1" class="DigNum (strict)" method="Reinit To Default"() -> ()  [unwired: 3 in, 3 out]
      n249 = invoke on="Det 6" class="DigNum (strict)" method="Reinit To Default"() -> ()  [unwired: 3 in, 3 out]
      n250 = invoke on="Det 2" class="DigNum (strict)" method="Reinit To Default"() -> ()  [unwired: 3 in, 3 out]
      n251 = invoke on="Det 7" class="DigNum (strict)" method="Reinit To Default"() -> ()  [unwired: 3 in, 3 out]
      n252 = invoke on="Det 3" class="DigNum (strict)" method="Reinit To Default"() -> ()  [unwired: 3 in, 3 out]
      n253 = invoke on="Det 8" class="DigNum (strict)" method="Reinit To Default"() -> ()  [unwired: 3 in, 3 out]
      n254 = invoke on="Det 4" class="DigNum (strict)" method="Reinit To Default"() -> ()  [unwired: 3 in, 3 out]
      n255 = invoke on="Time Left (ms)" class="DigNum (strict)" method="Reinit To Default"() -> ()  [unwired: 3 in, 3 out]
      n256 = invoke on="Trial #" class="DigNum (strict)" method="Reinit To Default"() -> ()  [unwired: 3 in, 3 out]
      n257 = invoke on="g2" class="XYGraph (strict)" method="Reinit To Default"() -> ()  [unwired: 3 in, 3 out]
      n258 = invoke on="Frame #" class="DigNum (strict)" method="Reinit To Default"() -> ()  [unwired: 3 in, 3 out]
      n259 = call "ReadInitialAverages.vi"() -> ("avgOut"=w274:bool[][])  [unwired: 11 in]
      n260 = Build Array(FALSE) -> (w271:bool[])
      n261 = Initialize Array(FALSE, 4) -> (w273:bool[])
      n262 = property on="Tau" class="WFChart (strict)"("History Data"=cluster{"tmp":dbl, dbl}[] []) -> ()  [unwired: 2 in, 2 out]
      n263 = property on="Avg" class="Arr (strict)"("Value"=w274) -> ()  [unwired: 2 in, 2 out]
      n264 = call "DAQ Assistant14"("data"=w271) -> ()  [unwired: 17 in, 2 out]
      n265 = property on="Visible Averages" class="Arr (strict)"("Value"=w273) -> ()  [unwired: 2 in, 2 out]
      n266 = Bundle(w275, w275, w275, w275, w275, w275, w275, w275, w275, w275, w275, w275) -> (w276:T6)  [unwired: 1 in]
      n267 = case shown="\"8 Detectors\", Default" "Detector Select" {
        tunnel: [TRUE FALSE] -> w281
        frame "4 Detectors" {
        }
        frame "8 Detectors", Default {
        }
      }
      n268 = Initialize Array(w276, w275) -> ()  [unwired: 1 out]
      n269 = local write "4CH?"(w281) -> ()
    }
    frame #1 {
      n270 = while {
        stop <- w287 stop-if-true
        # "Looks at whether using 4 or 8 ch correlator\nGenerates time points for g2 function based on correlator"
        n271 = local read "Detector Select"() -> (w284:enum32{"4 Detectors", "8 Detectors"})
        n272 = call "DelayTime.vi"("Detector Select"=w284) -> ("Delaytime"=w285:sgl[])
        n273 = event shown="[2] \"Sequence Scan\": Value Change" {
          selector: _ -> [_ _ _ _ _]
          dyn-events: _ -> [_ _ _ _ _]
          timeout: 500 -> [_ _ _ _ _]
          tunnel: w285 -> [_ _ w372 _ _]
          tunnel: [_ _ _ "QUIT" _] -> w287
          tunnel: w284 -> [_ w363 w368 w816 _]
          event Menu Selection (User) {
            n274 = event-data() -> ("ItemTag"=w288:string)  [unwired: 1 in, 6 out]
            n275 = case shown="\"Save Options As...\"" w288 {
              frame "Save Options As..." {
                n276 = call "File Dialog2"("prompt"="Save Options As...", "pattern (all files)"="*.opt", "pattern label"="Options File") -> ("selected path"=w290:path, "error out"=w289:errorcluster)  [unwired: 9 in, 2 out]
                n277 = case shown="No Error" w289 {
                  selector: w289 -> [w294 _]
                  tunnel: w290 -> [_ w325]
                  frame Error {
                    n278 = call <vilib>:"Clear Errors.vi"("error in (no error)"=w294) -> ()  [unwired: 5 in, 2 out]
                  }
                  frame No Error {
                    w312 = "Flow Options"
                    n279 = local read "Update Time (ms)\nDO NOT CHANGE!"() -> (w305:u32)
                    n280 = Get Date/Time In Seconds() -> (seconds since 1Jan1904=w311:timestamp)
                    n281 = Format Date/Time String(seconds (now)=w311) -> (date/time string=w307:string)  [unwired: 2 in]
                    n282 = call <vilib>:"Open Config Data.vi"("create file if necessary (T)"=TRUE, "configuration file path"=w325) -> ("error out"=w323:errorcluster, "refnum"=w322:T7)  [unwired: 7 in, 1 out]
                    n283 = local read "Integration Time (ms)"() -> (w303:sgl)
                    n284 = call-poly <vilib>:"Write Key.vi"("section"="File Info", "error in (no error)"=w323, "value"=w307, "key"="Options Saved Time", "refnum"=w322) -> ("error out"=w309:errorcluster, "refnum out"=w310:T7)  [unwired: 4 in, 1 out]
                    n285 = call-poly <vilib>:"Write Key.vi"("section"=w312, "error in (no error)"=w309, "value"=w305, "key"="Updated Time", "refnum"=w310) -> ("error out"=w321:errorcluster, "refnum out"=w320:T7)  [unwired: 4 in, 1 out]
                    n286 = local read "Source#"() -> (w302:u32)
                    n287 = call-poly <vilib>:"Write Key.vi"("section"=w312, "error in (no error)"=w321, "value"=w303, "key"="Duration Time", "refnum"=w320) -> ("error out"=w316:errorcluster, "refnum out"=w317:T7)  [unwired: 4 in, 1 out]
                    n288 = local read "Detector#"() -> (w299:u32)
                    n289 = call-poly <vilib>:"Write Key.vi"("section"=w312, "error in (no error)"=w316, "value"=w302, "key"="Source to Flow", "refnum"=w317) -> ("error out"=w318:errorcluster, "refnum out"=w319:T7)  [unwired: 4 in, 1 out]
                    n290 = local read "Detector Select"() -> (w297:enum32{"4 Detectors", "8 Detectors"})
                    n291 = call-poly <vilib>:"Write Key.vi"("section"=w312, "error in (no error)"=w318, "value"=w299, "key"="Detector to Flow", "refnum"=w319) -> ("error out"=w315:errorcluster, "refnum out"=w314:T7)  [unwired: 4 in, 1 out]
                    n292 = call-poly <vilib>:"Write Key.vi"("section"=w312, "error in (no error)"=w315, "value"=w297, "key"="Detector Select", "refnum"=w314) -> ("error out"=w295:errorcluster, "refnum out"=w296:T7)  [unwired: 4 in, 1 out]
                    n293 = call <vilib>:"Close Config Data.vi"("error in (no error)"=w295, "refnum"=w296) -> ()  [unwired: 8 in, 2 out]
                  }
                }
              }
              frame "Load Options From..." {
                n294 = call "File Dialog3"("prompt"="Load Options From...", "pattern (all files)"="*.opt", "pattern label"="Options File") -> ("selected path"=w327:path, "error out"=w326:errorcluster)  [unwired: 9 in, 2 out]
                n295 = case shown="No Error" w326 {
                  selector: w326 -> [_ w356]
                  tunnel: w327 -> [w331 _]
                  frame No Error {
                    w346 = "Flow Options"
                    n296 = call <vilib>:"Open Config Data.vi"("create file if necessary (T)"=FALSE, "configuration file path"=w331) -> ("error out"=w338:errorcluster, "refnum"=w337:T7)  [unwired: 7 in, 1 out]
                    n297 = call-poly <vilib>:"Read Key.vi"("section"=w346, "error in (no error)"=w338, "key"="Updated Time", "refnum"=w337) -> ("error out"=w354:errorcluster, "value"=w336:u32, "refnum out"=w353:T7)  [unwired: 4 in, 1 out]
                    n298 = local write "Update Time (ms)\nDO NOT CHANGE!"(w336) -> ()
                    n299 = call-poly <vilib>:"Read Key.vi"("section"=w346, "error in (no error)"=w354, "key"="Duration Time", "refnum"=w353) -> ("error out"=w349:errorcluster, "value"=w335:i32, "refnum out"=w350:T7)  [unwired: 4 in, 1 out]
                    n300 = local write "Integration Time (ms)"(w335) -> ()
                    n301 = call-poly <vilib>:"Read Key.vi"("section"=w346, "error in (no error)"=w349, "key"="Source to Flow", "refnum"=w350) -> ("error out"=w351:errorcluster, "value"=w332:u32, "refnum out"=w352:T7)  [unwired: 4 in, 1 out]
                    n302 = local write "Source#"(w332) -> ()
                    n303 = call-poly <vilib>:"Read Key.vi"("section"=w346, "error in (no error)"=w351, "key"="Detector to Flow", "refnum"=w352) -> ("error out"=w348:errorcluster, "value"=w333:u32, "refnum out"=w347:T7)  [unwired: 4 in, 1 out]
                    n304 = local write "Detector#"(w333) -> ()
                    n305 = call-poly <vilib>:"Read Key.vi"("section"=w346, "error in (no error)"=w348, "key"="Detector Select", "refnum"=w347) -> ("error out"=w339:errorcluster, "value"=w334:u32, "refnum out"=w340:T7)  [unwired: 4 in, 1 out]
                    n306 = call <vilib>:"Close Config Data.vi"("error in (no error)"=w339, "refnum"=w340) -> ()  [unwired: 8 in, 2 out]
                    n307 = local write "Detector Select"(w334) -> ()
                  }
                  frame Error {
                    n308 = call <vilib>:"Clear Errors.vi"("error in (no error)"=w356) -> ()  [unwired: 5 in, 2 out]
                  }
                }
              }
              frame "Plot Settings..." {
                # "This part is kind of weird right now. It seems that there are controls\nfor this but those things cannot be selected."
                n309 = local read "Detector#"() -> (w358:u32)
                n310 = local read "Source#"() -> (w359:u32)
                n311 = call "PlotSettings.vi"("Detectorin"=w358, "Sourcein"=w359) -> ("Detector#"=→"Detector#":u32, "Source#"=→"Source#":u32)
              }
              frame Default {
              }
            }
          }
          event "Initialize Correlator": Value Change {
            # "Initialize Correlator"
            n312 = event-data() -> ()  [unwired: 1 in, 5 out]
            n313 = case shown="\"8 Detectors\", Default" w363 {
              tunnel: [TRUE FALSE] -> w362
              frame "4 Detectors" {
              }
              frame "8 Detectors", Default {
              }
            }
            "4CH?" <- w362
            n314 = invoke on="Trial #" class="DigNum (strict)" method="Reinit To Default"() -> ()  [unwired: 3 in, 3 out]
            n315 = invoke on="Det 5" class="DigNum (strict)" method="Reinit To Default"() -> ()  [unwired: 3 in, 3 out]
            n316 = invoke on="g2" class="XYGraph (strict)" method="Reinit To Default"() -> ()  [unwired: 3 in, 3 out]
            n317 = invoke on="Det 1" class="DigNum (strict)" method="Reinit To Default"() -> ()  [unwired: 3 in, 3 out]
            n318 = invoke on="Det 2" class="DigNum (strict)" method="Reinit To Default"() -> ()  [unwired: 3 in, 3 out]
            n319 = invoke on="Det 6" class="DigNum (strict)" method="Reinit To Default"() -> ()  [unwired: 3 in, 3 out]
            n320 = invoke on="Frame #" class="DigNum (strict)" method="Reinit To Default"() -> ()  [unwired: 3 in, 3 out]
            n321 = invoke on="Det 3" class="DigNum (strict)" method="Reinit To Default"() -> ()  [unwired: 3 in, 3 out]
            n322 = invoke on="Det 7" class="DigNum (strict)" method="Reinit To Default"() -> ()  [unwired: 3 in, 3 out]
            n323 = invoke on="Det 4" class="DigNum (strict)" method="Reinit To Default"() -> ()  [unwired: 3 in, 3 out]
            n324 = invoke on="Det 8" class="DigNum (strict)" method="Reinit To Default"() -> ()  [unwired: 3 in, 3 out]
            n325 = invoke on="Time Left (ms)" class="DigNum (strict)" method="Reinit To Default"() -> ()  [unwired: 3 in, 3 out]
            n326 = invoke on="Mark #" class="DigNum (strict)" method="Reinit To Default"() -> ()  [unwired: 3 in, 3 out]
            n327 = property on="Tau" class="WFChart (strict)"("History Data"=cluster{"tmp":dbl, dbl}[] []) -> ()  [unwired: 2 in, 2 out]
          }
          event "Sequence Scan": Value Change {
            # "Initialize Baseline"
            n328 = event-data() -> ()  [unwired: 1 in, 6 out]
            n329 = case shown="\"8 Detectors\", Default" w368 {
              tunnel: [w811 w812] -> w367
              frame "4 Detectors" {
                n330 = local read "4CH?"() -> (w811:bool)
              }
              frame "8 Detectors", Default {
                # "Select whether using 4 or 8ch correlator"
                n331 = local read "4CH?"() -> (w813:bool)
                n332 = Not(x=w813) -> (.not. x?=w812:bool)
              }
            }
            n333 = case shown="True" w367 {
              selector: w367 -> [w374 _]
              tunnel: w372 -> [_ w388]
              tunnel: w368 -> [_ w389]
              tunnel: sgl 1.0 -> [_ w387]
              frame False {
                n334 = invoke on="Sequence Scan" class="Bool" method="Reinit To Default"() -> ()  [unwired: 3 in, 3 out]
                n335 = Not(x=w374) -> (.not. x?=w373:bool)
                n336 = call "Display Message to User3"("Enable"=w373, "Message"="ATTENTION:\nYou have changed Detector Select,\nplease press Initialize Correlator first!") -> ()  [unwired: 8 in, 2 out]
              }
              frame True {
                # "This part pauses and alerts user that test function is on. If test function is accepted then code runs but data is not saved (no timestamp either)."
                # "This checks for if the file already exists in the\ndirectory using the timing file. \n*If YES, then we don't do anything to the lasers. We just display message and wait for the user to input a new name and press sequence again.\n*If NO, then we proceed as per normal."
                n337 = case shown="False" "Test" {
                  selector: "Test" -> [w391 _]
                  tunnel: "Test" -> [_ w393]
                  tunnel: [w390 w392] -> w377
                  frame False {
                    n338 = Not(x=w391) -> (.not. x?=w390:bool)
                  }
                  frame True {
                    n339 = call "Test ON"("Enable"=w393) -> ("No - STOP"=w394:bool, "OK"=w392:bool)  [unwired: 15 in, 2 out]
                    n340 = local write "Stop"(w394) -> ()
                  }
                }
                n341 = local read "File Name:"() -> (w383:string)
                n342 = local read "Data Save Directory:"() -> (w382:path)
                n343 = Concatenate Strings(w383, "_TIMING", ".dat") -> (w385:string)
                n344 = Build Path(base path=w382, name or relative path=w385) -> (appended path=w381:path)
                n345 = call <vilib>:"Check if File or Folder Exists.vi"("path"=w381) -> ("file or folder exists?"=w379:bool)  [unwired: 8 in, 2 out]
                n346 = Not(x=w379) -> (.not. x?=w380:bool)
                n347 = Not And(1:w377, 2:w380) -> (0:w378:bool)
                n348 = case shown="False" w378 {
                  tunnel: w389 -> [w401 _]
                  tunnel: w388 -> [w400 _]
                  tunnel: w387 -> [w399 _]
                  frame False {
                    n349 = local read "Test"() -> (w397:bool)
                    n350 = case shown="False" w397 {
                      frame False {
                        # "This bit stores the time stamp."
                        n351 = local read "File Name:"() -> (w402:string)
                        n352 = local read "Data Save Directory:"() -> (w403:path)
                        n353 = Concatenate Strings(w402, "_TIMING", ".dat") -> (w407:string)
                        n354 = Get Date/Time In Seconds() -> (seconds since 1Jan1904=w404:timestamp)
                        n355 = Build Path(base path=w403, name or relative path=w407) -> (appended path=w406:path)
                        n356 = Format Date/Time String(seconds (now)=w404) -> (date/time string=w410:string)  [unwired: 2 in]
                        n357 = Write to Text File(file (use dialog)=w406, text=w410) -> (refnum out=w409:refnum<file>, error out=w408:errorcluster)  [unwired: 2 in, 1 out]
                        n358 = Close File(refnum=w409, error in=w408) -> ()  [unwired: 2 out]
                      }
                      frame True {
                      }
                    }
                    n359 = while {
                      tunnel: w401 -> [w445]
                      tunnel: w400 -> [w444]
                      tunnel: w399 -> [_]
                      stop <- w431 stop-if-true
                      (unwired) u32 11
                      (unwired) u32 9
                      (unwired) u32 10
                      (unwired) u32 8
                      # "Only runs Real Time Fitting if \nReal Time Fitting box is checked \nand test function is off."
                      # "After everything is done, we have to\nbe nice and turn off them lasers and\nreset all the buttons."
                      n360 = for {
                        N: 1 -> [_]
                        tunnel: w444 -> [w463]
                        tunnel: w445 -> [w462]
                        tunnel: [w459] -> w431
                        tunnel: [w458] -> w442
                        tunnel: [w457] -> w435
                        tunnel: [w456] -> w434
                        tunnel: [w455] -> w433
                        # "The logic here may look funny but it works elegantly. No matter if you choose \"Use Both Lasers\", the AND output is always\nfalse the first time these two boxes run since Laser 1 Value is always false, and the default is to use flow laser 1.\nBUT, the trick is if you chose \"Use Both Laser\" This big for loop is gonna run twice, the second time it runs, \nthe laser 1 value is TRUE because it is set to TRUE by the second box when the big for loop ran the first time. Now, when\nthe output of AND is true, ISS laser no longer runs. Only flow laser two is turned on and we execute the for loop to the right."
                        # "These two boxes take care of the flow chart.\nIt turn on ISS laser first, then triggers it and turn it off.\nIf ISS data is ready, then we go on to flow lase."
                        # "This loop may seem useless but it acts as a block. \nThis block does all the data collection, plotting and writing the data\nto file"
                        n361 = stacked-sequence {
                          tunnel: [_ _ _ _ _ _ w486] -> w454
                          frame #0 {
                            # "DCS LASER OFF"
                            # "Turn relay off so that Optical switch is closed and LED indicator is OFF"
                            n362 = Build Array(FALSE, FALSE) -> (w466:bool[])
                            n363 = call "DAQ Assistant9"("data"=w466) -> ()  [unwired: 17 in, 2 out]
                            n364 = call "iBs.vi"("Laser On/Off"=FALSE, "VISA resource name"="Laser Input Name") -> ()
                          }
                          frame #1 {
                            # "ISS lasers ON"
                            n365 = Wait (ms)(milliseconds to wait=u32 100) -> ()  [unwired: 1 out]
                            n366 = Build Array(TRUE) -> (w470:bool[])
                            n367 = call "DAQ Assistant10"("data"=w470) -> ()  [unwired: 17 in, 2 out]
                          }
                          frame #2 {
                            n368 = stacked-sequence {
                              frame #0 {
                                # "ISS Data TRIGGER"
                                n369 = Build Array(TRUE) -> (w473:bool[])
                                n370 = call "DAQ Assistant12"("data"=w473) -> ()  [unwired: 17 in, 2 out]
                              }
                              frame #1 {
                                n371 = Wait (ms)(milliseconds to wait=u32 1000) -> ()  [unwired: 1 out]
                              }
                            }
                          }
                          frame #3 {
                            # "Make sure a second trigger isnt caught by turning trigger signal LOW"
                            n372 = Build Array(FALSE) -> (w475:bool[])
                            n373 = call "DAQ Assistant13"("data"=w475) -> ()  [unwired: 17 in, 2 out]
                          }
                          frame #4 {
                            # "Wait for AQ Active signal from ISS to go LOW"
                            n374 = while {
                              stop <- w477 continue-if-true
                              # "Loop until Dig Input signal is false"
                              n375 = Wait Until Next ms Multiple(millisecond multiple=u32 100 ("milliseconds to wait")) -> ()  [unwired: 1 out]
                              n376 = call "DAQ Assistant7"() -> ("data"=w478:bool[])  [unwired: 17 in, 2 out]
                              n377 = And Array Elements(Boolean array=w478) -> (logical AND=w477:bool)
                            }
                          }
                          frame #5 {
                            # "ISS lasers OFF"
                            # "Wait 500ms and then move on"
                            n378 = while {
                              stop <- TRUE stop-if-true
                              n379 = Wait (ms)(milliseconds to wait=500) -> ()  [unwired: 1 out]
                            }
                            n380 = Build Array(FALSE) -> (w480:bool[])
                            n381 = call "DAQ Assistant"("data"=w480) -> ()  [unwired: 17 in, 2 out]
                          }
                          frame #6 {
                            # "DCS LASER ON"
                            # "Turn relay ON so that Optical switch is open and LED indicator is ON"
                            n382 = Build Array(TRUE, TRUE) -> (w487:bool[])
                            n383 = local read "Laser Input Name"() -> (w484:refnum<visa-resource-name>)
                            n384 = call "DAQ Assistant11"("data"=w487) -> ()  [unwired: 17 in, 2 out]
                            n385 = call "iBs.vi"("Laser On/Off"=TRUE, "VISA resource name"=w484) -> ()
                            n386 = while {
                              tunnel: [w490] -> w486
                              stop <- w490 stop-if-true
                              w490 = TRUE
                              n387 = Wait (ms)(milliseconds to wait=200) -> ()  [unwired: 1 out]
                            }
                          }
                        }
                        n388 = case shown="\"8 Detectors\", Default" w462 {
                          selector: w462 -> [w809 w810]
                          tunnel: [w809 w810] -> w460
                          tunnel: w454 -> [_ _]
                          frame "4 Detectors" {
                          }
                          frame "8 Detectors", Default {
                          }
                        }
                        n389 = for {
                          N: 1 -> [_]
                          tunnel: w463 -> [w512]
                          tunnel: [w496] -> w459
                          tunnel: w460 -> [w501]
                          tunnel: [w504] -> w458
                          tunnel: "MARK\nMark" -> [w503]
                          tunnel: [w502] -> w457
                          tunnel: [w494] -> w456
                          tunnel: [w500] -> w455
                          w513 = FALSE
                          w522 = u8 2
                          # "Only saves data if\ntest function is off."
                          # "If Fixed # Frames check box is selected,\ncode will run for # of frames specified on \nfront panel and then call Stop button"
                          # "This for loop here acts as a block as well. It takes the relative \nflow data from UpdateData.vi and plot the data on the graph.\nWhen \"Baseline\" is selected,  the data point goes to 1. When\n\"Mark\" is selected, a point at positive infinity is plotted and a\nvertical line joining the point and the x axis if displayed."
                          n390 = while {
                            tunnel: [w693] -> w521
                            tunnel: [w694] -> w520
                            tunnel: [w667] -> w519
                            tunnel: [w665] -> w496
                            tunnel: [w695] -> w518
                            tunnel: w512 -> [w697]
                            tunnel: w501 -> [w668]
                            stop <- w700 stop-if-true
                            n391 = Not(x="D3") -> (.not. x?=w682:bool)
                            n392 = Not(x="D4") -> (.not. x?=w681:bool)
                            n393 = Not(x="D8") -> (.not. x?=w677:bool)
                            n394 = Not(x="D5") -> (.not. x?=w680:bool)
                            n395 = Not(x="D1") -> (.not. x?=w684:bool)
                            n396 = Not(x="D6") -> (.not. x?=w679:bool)
                            n397 = Not(x="D2") -> (.not. x?=w669:bool)
                            n398 = Not(x="D7") -> (.not. x?=w678:bool)
                            n399 = case shown="True" "Stop" {
                              selector: "Stop" -> [w739 w746]
                              tunnel: [w739 w743] -> w665
                              frame False {
                              }
                              frame True {
                                # "Turn relay off so that Optical switch is closed and LED indicator is OFF"
                                n400 = call "Prompt User for Input"("Enable"=w746) -> ("Yes"=w743:bool)  [unwired: 17 in, 1 out]
                                n401 = local read "Laser Input Name"() -> (w740:refnum<visa-resource-name>)
                                n402 = Not(x=w743) -> (.not. x?=w742:bool)
                                n403 = Build Array(w742, FALSE) -> (w745:bool[])
                                n404 = call "DAQ Assistant2"("data"=w745) -> ()  [unwired: 17 in, 2 out]
                                n405 = call "iBs.vi"("Laser On/Off"=FALSE, "VISA resource name"=w740) -> ()
                              }
                            }
                            n406 = case shown="True" "Clear plots" {
                              frame False {
                              }
                              frame True {
                                n407 = invoke on="g2" class="XYGraph (strict)" method="Reinit To Default"() -> ()  [unwired: 3 in, 3 out]
                                n408 = property on="Tau" class="WFChart (strict)"("History Data"=cluster{"tmp":dbl, dbl}[] []) -> ()  [unwired: 2 in, 2 out]
                              }
                            }
                            n409 = case shown="True" w682 {
                              selector: w682 -> [w779 w780]
                              frame False {
                                n410 = property on="g2" class="XYGraph (strict)"("Active Plot"=u32 2) -> (error out=w777:errorcluster)  [unwired: 2 in, 1 out]
                                n411 = property on="g2" class="XYGraph (strict)"(error in=w777, "Plot.Visible?"=w779) -> ()  [unwired: 1 in, 2 out]
                              }
                              frame True {
                                (unwired) u32 2
                                n412 = property on="g2" class="XYGraph (strict)"("Active Plot"=u32 2) -> (error out=w781:errorcluster)  [unwired: 2 in, 1 out]
                                n413 = property on="g2" class="XYGraph (strict)"(error in=w781, "Plot.Visible?"=w780) -> ()  [unwired: 1 in, 2 out]
                              }
                            }
                            n414 = case shown="True" w681 {
                              selector: w681 -> [w773 w774]
                              frame False {
                                n415 = property on="g2" class="XYGraph (strict)"("Active Plot"=u32 3) -> (error out=w771:errorcluster)  [unwired: 2 in, 1 out]
                                n416 = property on="g2" class="XYGraph (strict)"(error in=w771, "Plot.Visible?"=w773) -> ()  [unwired: 1 in, 2 out]
                              }
                              frame True {
                                (unwired) u32 3
                                n417 = property on="g2" class="XYGraph (strict)"("Active Plot"=u32 3) -> (error out=w775:errorcluster)  [unwired: 2 in, 1 out]
                                n418 = property on="g2" class="XYGraph (strict)"(error in=w775, "Plot.Visible?"=w774) -> ()  [unwired: 1 in, 2 out]
                              }
                            }
                            n419 = case shown="True" w677 {
                              selector: w677 -> [w749 w750]
                              frame False {
                                n420 = property on="g2" class="XYGraph (strict)"("Active Plot"=u32 7) -> (error out=w747:errorcluster)  [unwired: 2 in, 1 out]
                                n421 = property on="g2" class="XYGraph (strict)"(error in=w747, "Plot.Visible?"=w749) -> ()  [unwired: 1 in, 2 out]
                              }
                              frame True {
                                (unwired) u32 7
                                n422 = property on="g2" class="XYGraph (strict)"("Active Plot"=u32 7) -> (error out=w751:errorcluster)  [unwired: 2 in, 1 out]
                                n423 = property on="g2" class="XYGraph (strict)"(error in=w751, "Plot.Visible?"=w750) -> ()  [unwired: 1 in, 2 out]
                              }
                            }
                            n424 = case shown="True" w680 {
                              selector: w680 -> [w767 w768]
                              frame False {
                                n425 = property on="g2" class="XYGraph (strict)"("Active Plot"=u32 4) -> (error out=w765:errorcluster)  [unwired: 2 in, 1 out]
                                n426 = property on="g2" class="XYGraph (strict)"(error in=w765, "Plot.Visible?"=w767) -> ()  [unwired: 1 in, 2 out]
                              }
                              frame True {
                                (unwired) u32 4
                                n427 = property on="g2" class="XYGraph (strict)"("Active Plot"=u32 4) -> (error out=w769:errorcluster)  [unwired: 2 in, 1 out]
                                n428 = property on="g2" class="XYGraph (strict)"(error in=w769, "Plot.Visible?"=w768) -> ()  [unwired: 1 in, 2 out]
                              }
                            }
                            n429 = case shown="True" w684 {
                              selector: w684 -> [w792 w793]
                              frame False {
                                n430 = property on="g2" class="XYGraph (strict)"("Active Plot"=u32 0) -> (error out=w790:errorcluster)  [unwired: 2 in, 1 out]
                                n431 = property on="g2" class="XYGraph (strict)"(error in=w790, "Plot.Visible?"=w792) -> ()  [unwired: 1 in, 2 out]
                              }
                              frame True {
                                (unwired) u32 0
                                n432 = property on="g2" class="XYGraph (strict)"("Active Plot"=u32 0) -> (error out=w794:errorcluster)  [unwired: 2 in, 1 out]
                                n433 = property on="g2" class="XYGraph (strict)"(error in=w794, "Plot.Visible?"=w793) -> ()  [unwired: 1 in, 2 out]
                              }
                            }
                            n434 = case shown="True" w679 {
                              selector: w679 -> [w761 w762]
                              frame False {
                                n435 = property on="g2" class="XYGraph (strict)"("Active Plot"=u32 5) -> (error out=w759:errorcluster)  [unwired: 2 in, 1 out]
                                n436 = property on="g2" class="XYGraph (strict)"(error in=w759, "Plot.Visible?"=w761) -> ()  [unwired: 1 in, 2 out]
                              }
                              frame True {
                                (unwired) u32 5
                                n437 = property on="g2" class="XYGraph (strict)"("Active Plot"=u32 5) -> (error out=w763:errorcluster)  [unwired: 2 in, 1 out]
                                n438 = property on="g2" class="XYGraph (strict)"(error in=w763, "Plot.Visible?"=w762) -> ()  [unwired: 1 in, 2 out]
                              }
                            }
                            n439 = case shown="True" w669 {
                              selector: w669 -> [w785 w786]
                              frame False {
                                n440 = property on="g2" class="XYGraph (strict)"("Active Plot"=u32 1) -> (error out=w783:errorcluster)  [unwired: 2 in, 1 out]
                                n441 = property on="g2" class="XYGraph (strict)"(error in=w783, "Plot.Visible?"=w785) -> ()  [unwired: 1 in, 2 out]
                              }
                              frame True {
                                (unwired) u32 1
                                n442 = property on="g2" class="XYGraph (strict)"("Active Plot"=u32 1) -> (error out=w787:errorcluster)  [unwired: 2 in, 1 out]
                                n443 = property on="g2" class="XYGraph (strict)"(error in=w787, "Plot.Visible?"=w786) -> ()  [unwired: 1 in, 2 out]
                              }
                            }
                            n444 = case shown="True" w678 {
                              selector: w678 -> [w755 w756]
                              frame False {
                                n445 = property on="g2" class="XYGraph (strict)"("Active Plot"=u32 6) -> (error out=w753:errorcluster)  [unwired: 2 in, 1 out]
                                n446 = property on="g2" class="XYGraph (strict)"(error in=w753, "Plot.Visible?"=w755) -> ()  [unwired: 1 in, 2 out]
                              }
                              frame True {
                                (unwired) u32 6
                                n447 = property on="g2" class="XYGraph (strict)"("Active Plot"=u32 6) -> (error out=w757:errorcluster)  [unwired: 2 in, 1 out]
                                n448 = property on="g2" class="XYGraph (strict)"(error in=w757, "Plot.Visible?"=w756) -> ()  [unwired: 1 in, 2 out]
                              }
                            }
                            n449 = call "UpdateData.vi"("Duration Time (ms)"="Integration Time (ms)", "Detector Select"=w668, "Delay Time"=w697) -> ("Elapsed Time(s)"=w699:sgl, "Intensity Array"=w696:sgl[], "Tau Array"=w695:sgl[], "Intensity data"=w693:string, "g2 Display"=→"g2":cluster{"Delay Time":sgl[], sgl[]}[], "tau data"=w694:string, "g2 data"=w667:string)  [unwired: 2 in, 8 out]
                            n450 = Wait (ms)(milliseconds to wait="Update Time (ms)\nDO NOT CHANGE!") -> ()  [unwired: 1 out]
                            n451 = Multiply(x=sgl 1000.0, y=w699) -> (x*y=w703:sgl)
                            n452 = Index Array(array=w696, index #1=0, index #2=1, index #3=2, index #4=3, index #5=4, index #6=5, index #7=6, index #8=7) -> (element #1=w599:sgl, element #2=w598:sgl, element #3=w597:sgl, element #4=w596:sgl, element #5=w595:sgl, element #6=w594:sgl, element #7=w593:sgl, element #8=w592:sgl)
                            "Det 7" <- w593
                            "Det 6" <- w594
                            "Det 5" <- w595
                            "Det 4" <- w596
                            "Det 3" <- w597
                            "Det 2" <- w598
                            "Det 1" <- w599
                            "Det 8" <- w592
                            n453 = Subtract(x="Integration Time (ms)", y=w703) -> (x-y=w701:sgl)
                            "Time Left (ms)" <- w701
                            n454 = Greater Or Equal?(x=w599, y=sgl 2.0) -> (x >= y?=w661:bool)
                            n455 = Greater Or Equal?(x=w598, y=sgl 2.0) -> (x >= y?=w656:bool)
                            n456 = Greater Or Equal?(x=w597, y=sgl 2.0) -> (x >= y?=w651:bool)
                            n457 = Greater Or Equal?(x=w596, y=sgl 2.0) -> (x >= y?=w646:bool)
                            n458 = Greater?(x=w599, y=0.98) -> (0:w577:bool)
                            n459 = Greater?(x=w598, y=0.98) -> (0:w579:bool)
                            n460 = Greater?(x=w597, y=0.98) -> (0:w581:bool)
                            n461 = Greater?(x=w596, y=0.98) -> (0:w583:bool)
                            n462 = Less Or Equal?(x=w599, y=sgl 1000.0) -> (x <= y?=w662:bool)
                            n463 = Less Or Equal?(x=w598, y=sgl 1000.0) -> (x <= y?=w655:bool)
                            n464 = Less Or Equal?(x=w597, y=sgl 1000.0) -> (x <= y?=w650:bool)
                            n465 = Less Or Equal?(x=w596, y=sgl 1000.0) -> (x <= y?=w645:bool)
                            n466 = Less Or Equal?(x=w595, y=sgl 1000.0) -> (x <= y?=w640:bool)
                            n467 = Less Or Equal?(x=w594, y=sgl 1000.0) -> (x <= y?=w635:bool)
                            n468 = Less Or Equal?(x=w593, y=sgl 1000.0) -> (x <= y?=w630:bool)
                            n469 = Less Or Equal?(x=w592, y=sgl 1000.0) -> (x <= y?=w625:bool)
                            n470 = Less?(x=w599, y=1.005) -> (x < y?=w576:bool)
                            n471 = Less?(x=w598, y=1.005) -> (x < y?=w578:bool)
                            n472 = Less?(x=w597, y=1.005) -> (x < y?=w580:bool)
                            n473 = Less?(x=w596, y=1.005) -> (x < y?=w582:bool)
                            n474 = Less?(x=w595, y=1.005) -> (x < y?=w584:bool)
                            n475 = Less?(x=w594, y=1.005) -> (x < y?=w586:bool)
                            n476 = Less?(x=w593, y=1.005) -> (x < y?=w588:bool)
                            n477 = Less?(x=w592, y=1.005) -> (x < y?=w590:bool)
                            n478 = Greater Or Equal?(x=w595, y=sgl 2.0) -> (x >= y?=w641:bool)
                            n479 = Greater Or Equal?(x=w594, y=sgl 2.0) -> (x >= y?=w636:bool)
                            n480 = Greater Or Equal?(x=w593, y=sgl 2.0) -> (x >= y?=w631:bool)
                            n481 = Greater Or Equal?(x=w592, y=sgl 2.0) -> (x >= y?=w626:bool)
                            n482 = Greater?(x=w595, y=0.98) -> (0:w585:bool)
                            n483 = Greater?(x=w594, y=0.98) -> (0:w587:bool)
                            n484 = Greater?(x=w593, y=0.98) -> (0:w589:bool)
                            n485 = Greater?(x=w592, y=0.98) -> (0:w591:bool)
                            n486 = Build Array(w576, w577, w661, w662) -> (w663:bool[])
                            n487 = Build Array(w579, w578, w656, w655) -> (w654:bool[])
                            n488 = Build Array(w580, w581, w651, w650) -> (w649:bool[])
                            n489 = Build Array(w583, w582, w646, w645) -> (w644:bool[])
                            n490 = Build Array(w585, w584, w641, w640) -> (w639:bool[])
                            n491 = Build Array(w587, w586, w636, w635) -> (w634:bool[])
                            n492 = Build Array(w589, w588, w631, w630) -> (w629:bool[])
                            n493 = Build Array(w590, w591, w626, w625) -> (w624:bool[])
                            n494 = And Array Elements(Boolean array=w663) -> (logical AND=w623:bool)
                            n495 = And Array Elements(Boolean array=w654) -> (logical AND=w622:bool)
                            n496 = And Array Elements(Boolean array=w649) -> (logical AND=w621:bool)
                            n497 = And Array Elements(Boolean array=w644) -> (logical AND=w620:bool)
                            n498 = And Array Elements(Boolean array=w639) -> (logical AND=w619:bool)
                            n499 = And Array Elements(Boolean array=w634) -> (logical AND=w618:bool)
                            n500 = And Array Elements(Boolean array=w629) -> (logical AND=w617:bool)
                            n501 = And Array Elements(Boolean array=w624) -> (logical AND=w616:bool)
                            n502 = Less Or Equal To 0?(x=w701) -> (x <= 0?=w702:bool)
                            n503 = case shown="False" w623 {
                              frame False {
                                n504 = control-ref of="Det 1"() -> (w735:refnum<vi>)
                                n505 = property on="Property Node" class="Digital (strict)"(reference=w735, "DisabledEnum"=T5."Disabled and Grayed Out" ("Disabled")) -> ()  [unwired: 1 in, 2 out]
                              }
                              frame True {
                                n506 = control-ref of="Det 1"() -> (w737:refnum<vi>)
                                n507 = property on="Property Node" class="Digital (strict)"(reference=w737, "DisabledEnum"=T5."Enabled" ("Disabled")) -> ()  [unwired: 1 in, 2 out]
                              }
                            }
                            n508 = case shown="False" w622 {
                              frame False {
                                n509 = control-ref of="Det 2"() -> (w731:refnum<vi>)
                                n510 = property on="Property Node" class="Digital (strict)"(reference=w731, "DisabledEnum"=T5."Disabled and Grayed Out" ("Disabled")) -> ()  [unwired: 1 in, 2 out]
                              }
                              frame True {
                                n511 = control-ref of="Det 2"() -> (w733:refnum<vi>)
                                n512 = property on="Property Node" class="Digital (strict)"(reference=w733, "DisabledEnum"=T5."Enabled" ("Disabled")) -> ()  [unwired: 1 in, 2 out]
                              }
                            }
                            n513 = case shown="False" w621 {
                              frame False {
                                n514 = control-ref of="Det 3"() -> (w727:refnum<vi>)
                                n515 = property on="Property Node" class="Digital (strict)"(reference=w727, "DisabledEnum"=T5."Disabled and Grayed Out" ("Disabled")) -> ()  [unwired: 1 in, 2 out]
                              }
                              frame True {
                                n516 = control-ref of="Det 3"() -> (w729:refnum<vi>)
                                n517 = property on="Property Node" class="Digital (strict)"(reference=w729, "DisabledEnum"=T5."Enabled" ("Disabled")) -> ()  [unwired: 1 in, 2 out]
                              }
                            }
                            n518 = case shown="False" w620 {
                              frame False {
                                n519 = control-ref of="Det 4"() -> (w723:refnum<vi>)
                                n520 = property on="Property Node" class="Digital (strict)"(reference=w723, "DisabledEnum"=T5."Disabled and Grayed Out" ("Disabled")) -> ()  [unwired: 1 in, 2 out]
                              }
                              frame True {
                                n521 = control-ref of="Det 4"() -> (w725:refnum<vi>)
                                n522 = property on="Property Node" class="Digital (strict)"(reference=w725, "DisabledEnum"=T5."Enabled" ("Disabled")) -> ()  [unwired: 1 in, 2 out]
                              }
                            }
                            n523 = case shown="False" w619 {
                              frame False {
                                n524 = control-ref of="Det 5"() -> (w719:refnum<vi>)
                                n525 = property on="Property Node" class="Digital (strict)"(reference=w719, "DisabledEnum"=T5."Disabled and Grayed Out" ("Disabled")) -> ()  [unwired: 1 in, 2 out]
                              }
                              frame True {
                                n526 = control-ref of="Det 5"() -> (w721:refnum<vi>)
                                n527 = property on="Property Node" class="Digital (strict)"(reference=w721, "DisabledEnum"=T5."Enabled" ("Disabled")) -> ()  [unwired: 1 in, 2 out]
                              }
                            }
                            n528 = case shown="True" w618 {
                              frame False {
                                n529 = control-ref of="Det 6"() -> (w715:refnum<vi>)
                                n530 = property on="Property Node" class="Digital (strict)"(reference=w715, "DisabledEnum"=T5."Disabled and Grayed Out" ("Disabled")) -> ()  [unwired: 1 in, 2 out]
                              }
                              frame True {
                                n531 = control-ref of="Det 6"() -> (w717:refnum<vi>)
                                n532 = property on="Property Node" class="Digital (strict)"(reference=w717, "DisabledEnum"=T5."Enabled" ("Disabled")) -> ()  [unwired: 1 in, 2 out]
                              }
                            }
                            n533 = case shown="True" w617 {
                              frame False {
                                n534 = control-ref of="Det 7"() -> (w711:refnum<vi>)
                                n535 = property on="Property Node" class="Digital (strict)"(reference=w711, "DisabledEnum"=T5."Disabled and Grayed Out" ("Disabled")) -> ()  [unwired: 1 in, 2 out]
                              }
                              frame True {
                                n536 = control-ref of="Det 7"() -> (w713:refnum<vi>)
                                n537 = property on="Property Node" class="Digital (strict)"(reference=w713, "DisabledEnum"=T5."Enabled" ("Disabled")) -> ()  [unwired: 1 in, 2 out]
                              }
                            }
                            n538 = case shown="True" w616 {
                              frame False {
                                n539 = control-ref of="Det 8"() -> (w707:refnum<vi>)
                                n540 = property on="Property Node" class="Digital (strict)"(reference=w707, "DisabledEnum"=T5."Disabled and Grayed Out" ("Disabled")) -> ()  [unwired: 1 in, 2 out]
                              }
                              frame True {
                                n541 = control-ref of="Det 8"() -> (w709:refnum<vi>)
                                n542 = property on="Property Node" class="Digital (strict)"(reference=w709, "DisabledEnum"=T5."Enabled" ("Disabled")) -> ()  [unwired: 1 in, 2 out]
                              }
                            }
                            n543 = Or(x=w665, y=w702) -> (x .or. y?=w700:bool)
                            n544 = case shown="True" w700 {
                              tunnel: w668 -> [w796 _]
                              frame True {
                                n545 = case shown="\"8 Detectors\", Default" w796 {
                                frame "4 Detectors" {
                                }
                                frame "8 Detectors", Default {
                                }
                                }
                              }
                              frame False {
                              }
                            }
                          }
                          n546 = Current VI's Menubar() -> (w515:refnum<k9>)
                          n547 = local read "Trial #"() -> (w508:u32)
                          n548 = property on="QUIT" class="Bool"("Disabled"=w522) -> ()  [unwired: 2 in, 2 out]
                          n549 = Set Menu Item Info(7:"File", 9:w513, 11:w515) -> (3:w514:refnum<k9>)  [unwired: 4 in, 1 out]
                          n550 = Increment(x=w508) -> (x+1=w507:u32)
                          n551 = property on="Sequence Scan" class="Bool"("Disabled"=w522) -> ()  [unwired: 2 in, 2 out]
                          n552 = property on="Update Time (ms)\nDO NOT CHANGE!" class="DigNum (strict)"("Disabled"=w522) -> ()  [unwired: 2 in, 2 out]
                          n553 = property on="Integration Time (ms)" class="DigNum (strict)"("Disabled"=w522) -> ()  [unwired: 2 in, 2 out]
                          n554 = property on="Detector Select" class="RadioBtnsControl (strict)"("Disabled"=w522) -> ()  [unwired: 2 in, 2 out]
                          n555 = property on="Initialize Correlator" class="Bool"("Disabled"=w522) -> ()  [unwired: 2 in, 2 out]
                          n556 = local write "Trial #"(w507) -> ()
                          n557 = Set Menu Item Info(7:"Options", 9:w513, 11:w514) -> ()  [unwired: 4 in, 2 out]
                          n558 = case shown="\"Det 2\"" "Detector Used" {
                            tunnel: [1 2 3 4 5 6 7 8] -> w510
                            frame "Det 1", Default {
                            }
                            frame "Det 2" {
                            }
                            frame "Det 3" {
                            }
                            frame "Det 4" {
                            }
                            frame "Det 5" {
                            }
                            frame "Det 6" {
                            }
                            frame "Det 7" {
                            }
                            frame "Det 8" {
                            }
                          }
                          n559 = for {
                            N: 1 -> [_]
                            tunnel: w518 -> [w564]
                            tunnel: [w567] -> w511
                            tunnel: w510 -> [w566]
                            tunnel: w503 -> [w557]
                            n560 = case shown="True" w557 {
                              tunnel: [u32 0 w573] -> w567
                              frame False {
                              }
                              frame True {
                                n561 = local write "Trial #"(u32 0) -> ()
                                n562 = local read "Mark #"() -> (w575:u32)
                                n563 = Increment(x=w575) -> (x+1=w573:u32)
                                n564 = local write "Mark #"(w573) -> ()
                              }
                            }
                            n565 = Index Array(array=w564, index=w566) -> (element=w565:sgl)
                            n566 = Boolean To (0,1)(Boolean="Baseline") -> (0, 1=w569:i16)
                            n567 = case shown="False" w557 {
                              tunnel: [0.0 w571] -> w561
                              tunnel: inf -> [_ w571]
                              frame False {
                              }
                              frame True {
                              }
                            }
                            n568 = feedback #1() -> (w562:sgl)  [unwired: 1 in]
                            n569 = formula code="if(Tau==0) Tau=Tau+0.001;\nif(T==1) baselineflow=Tau;\n\ntmp=baselineflow/Tau;"("Tau"=w565, "T"=w569, "baselineflow"=w562) -> ("tmp"=w559:dbl, "baselineflow"=w563:sgl)
                            n570 = feedback-in #1(w563) -> ()
                            n571 = Bundle("tmp"=w559, w561) -> (→"Tau":cluster{"tmp":dbl, dbl})  [unwired: 1 in]
                          }
                          n572 = case shown="\"8 Detectors\", Default" w501 {
                            tunnel: w511 -> [w804 w808]
                            tunnel: [w805 w807] -> w528
                            tunnel: [4 8] -> w500
                            frame "4 Detectors" {
                              n573 = Build Array(w804, w804, w804, w804, w804) -> (w805:u32[])
                            }
                            frame "8 Detectors", Default {
                              n574 = Build Array(w808, w808, w808, w808, w808, w808, w808, w808, w808) -> (w807:u32[])
                            }
                          }
                          n575 = case shown="\"8 Detectors\", Default" w501 {
                            tunnel: ["%Duration\tID1\t\tID2\t\tID3\t\tID4\n" "%Duration\tID1\t\tID2\t\tID3\t\tID4\t\tID5\t\tID6\t\tID7\t\tID8\n"] -> w525
                            tunnel: ["%Tau\t\tTau1\t\tTau2\t\tTau3\t\tTau4\n" "%Tau\t\tTau1\t\tTau2\t\tTau3\t\tTau4\t\tTau5\t\tTau6\t\tTau7\t\tTau8\n"] -> w524
                            tunnel: ["%Delaytime\tD1\t\tD2\t\tD3\t\tD4\n" "%Delaytime\tD1\t\tD2\t\tD3\t\tD4\t\tD5\t\tD6\t\tD7\t\tD8\n"] -> w523
                            frame "4 Detectors" {
                            }
                            frame "8 Detectors", Default {
                            }
                          }
                          n576 = property on="Frame #" class="DigNum (strict)"() -> ("Value"=w494:u32)  [unwired: 2 in, 2 out]
                          n577 = case shown="True" "Fixed Time" {
                            tunnel: w494 -> [_ w548]
                            tunnel: [_ w545] -> w493
                            frame False {
                            }
                            frame True {
                              n578 = Increment(x="Fixed # of Frames") -> (x+1=w547:u32)
                              n579 = Less Or Equal?(x=w547, y=w548) -> (x <= y?=w545:bool)
                            }
                          }
                          n580 = Increment(x=w494) -> (x+1=w495:u32)
                          n581 = Number To Decimal String(number=w494) -> (decimal integer string=w529:string)  [unwired: 1 in]
                          n582 = Get Date/Time In Seconds() -> (seconds since 1Jan1904=w538:timestamp)
                          n583 = local write "Frame #"(w495) -> ()
                          n584 = Array To Spreadsheet String(array=w528, 3:"%d") -> (spreadsheet string=w526:string)  [unwired: 1 in]
                          n585 = Format Date/Time String(seconds (now)=w538) -> (date/time string=w535:string)  [unwired: 2 in]
                          "Computer Time" <- w535
                          n586 = Concatenate Strings("File Name:", "_flow_", w529, ".dat") -> (w498:string)
                          n587 = Concatenate Strings("%", w535, "\r\n", w525, w521, w524, "%\t\t", w520, w523, w519, w526) -> (w506:string)
                          n588 = Build Path(base path="Data Save Directory:", name or relative path=w498) -> (appended path=w505:path)
                          n589 = local read "Test"() -> (w492:bool)
                          n590 = case shown="False" w492 {
                            tunnel: w506 -> [w542 _]
                            tunnel: w505 -> [w541 _]
                            tunnel: [w540 _] -> w504
                            tunnel: [w539 _] -> w502
                            frame False {
                              n591 = Write to Text File(file (use dialog)=w541, text=w542) -> (refnum out=w543:refnum<file>, error out=w544:errorcluster)  [unwired: 2 in, 1 out]
                              n592 = Close File(refnum=w543, error in=w544) -> (path=w540:path, error out=w539:errorcluster)
                            }
                            frame True {
                            }
                          }
                          n593 = local write "Stop"(w493) -> ()
                        }
                      }
                      n594 = Index Array(array="Visible Averages", index=3) -> ()  [unwired: 1 out]
                      n595 = Index Array(array="Visible Averages", index=1) -> ()  [unwired: 1 out]
                      n596 = Index Array(array="Visible Averages", index=0) -> ()  [unwired: 1 out]
                      n597 = Index Array(array="Visible Averages", index=2) -> ()  [unwired: 1 out]
                      n598 = for {
                        N: 1 -> [_]
                        tunnel: w442 -> [_]
                        # "Turn relay off so that Optical switch is closed and LED indicator is OFF"
                        n599 = Build Array(FALSE, FALSE) -> (w449:bool[])
                        n600 = local read "Laser Input Name"() -> (w446:refnum<visa-resource-name>)
                        n601 = local write "Stop"(FALSE) -> ()
                        n602 = call "DAQ Assistant8"("data"=w449) -> ()  [unwired: 17 in, 2 out]
                        n603 = call "iBs.vi"("Laser On/Off"=FALSE, "VISA resource name"=w446) -> ()
                        n604 = Wait (ms)(milliseconds to wait="Delay between frames(ms)") -> ()  [unwired: 1 out]
                      }
                      n605 = Unbundle By Name(w435) -> ("status"=w441:bool)
                      n606 = local read "Test"() -> (w430:bool)
                      n607 = Not(x=w430) -> (.not. x?=w427:bool)
                      n608 = Not(x=w441) -> (.not. x?=w429:bool)
                      n609 = And(x="Real Time Fitting?", y=w427) -> (x .and. y?=w426:bool)
                      n610 = case shown="True" w426 {
                        tunnel: w429 -> [_ _]
                        tunnel: w434 -> [_ _]
                        tunnel: w433 -> [_ _]
                        frame False {
                        }
                        frame True {
                        }
                      }
                    }
                    n611 = case shown="True" "Record MAP data?" {
                      frame False {
                      }
                      frame True {
                        n612 = while {
                          stop <- w425 stop-if-true
                          n613 = local read "File Name:"() -> (w420:string)
                          n614 = local read "Data Save Directory:"() -> (w424:path)
                          n615 = Concatenate Strings(w420, "_MAP") -> (w423:string)
                          n616 = call "DAQ Assistant15"("rate"="Sampling Rate (Hz)", "number of samples"="Number Samples", "device name"="ExternalADC") -> ("data"=w417:dynamicdata, "error out"=w412:errorcluster)  [unwired: 13 in, 2 out]
                          "NIBP Data (*scaled by 98 to convert from V to mmHg)" <- w417
                          n617 = local read "Mark #"() -> (w418:u32)
                          n618 = Merge Signals(w417, w418) -> (w419:dynamicdata)
                          n619 = Build Path(base path=w424, name or relative path=w423) -> (appended path=w422:path)
                          n620 = call "Write To Measurement File"("Signals"=w419, "error in (no error)"=w412, "Filename"=w422) -> ("error out"=w413:errorcluster)  [unwired: 14 in, 2 out]
                          n621 = call <vilib>:"Clear Errors.vi"("error in (no error)"=w413) -> ()  [unwired: 5 in, 2 out]
                          n622 = local read "Stop"() -> (w425:bool)
                        }
                      }
                    }
                    n623 = local read "Fixed # of Frames"() -> (w396:u32)
                    n624 = Initialize Array(nan, w396) -> ()  [unwired: 1 out]
                  }
                  frame True {
                    n625 = invoke on="Sequence Scan" class="Bool" method="Reinit To Default"() -> ()  [unwired: 3 in, 3 out]
                    n626 = call "Display Message to User5"() -> ()  [unwired: 10 in, 2 out]
                  }
                }
              }
            }
            "Frame #" <- u32 0
            "Mark #" <- u32 0
            "Trial #" <- u32 0
          }
          event "QUIT": Value Change {
            # "Reset correlator before quitting"
            n627 = event-data() -> ()  [unwired: 1 in, 6 out]
            n628 = case shown="\"8 Detectors\", Default" w816 {
              frame "4 Detectors" {
              }
              frame "8 Detectors", Default {
              }
            }
            n629 = local write "Status"("Quit") -> ()
            n630 = local write "Status"("Quit") -> ()
          }
          event Timeout {
            w822 = TRUE
            w821 = u8 0
            # "This case structure turns on\n      and off the ISS Lasers"
            # "This case structure ensures that when the\noptical switch is turned on, the relay tells \nthe laser to power on."
            # "The system sits here and wait for some buttons to be pressed. And the status is always \"waiting\". Once some button is pressed, this value driven event\nstructure goes to the appropriate frame."
            n631 = event-data() -> ()  [unwired: 1 in, 3 out]
            n632 = local write "Status"("Waiting") -> ()
            n633 = property on="MARK\nMark" class="Bool"("DisabledEnum"=w821) -> ()  [unwired: 2 in, 2 out]
            n634 = property on="QUIT" class="Bool"("Disabled"=w821) -> ()  [unwired: 2 in, 2 out]
            n635 = property on="Sequence Scan" class="Bool"("Disabled"=w821) -> ()  [unwired: 2 in, 2 out]
            n636 = property on="Initialize Correlator" class="Bool"("Disabled"=w821) -> ()  [unwired: 2 in, 2 out]
            n637 = property on="Update Time (ms)\nDO NOT CHANGE!" class="DigNum (strict)"("Disabled"=w821) -> ()  [unwired: 2 in, 2 out]
            n638 = property on="Integration Time (ms)" class="DigNum (strict)"("Disabled"=w821) -> ()  [unwired: 2 in, 2 out]
            n639 = property on="Detector Select" class="RadioBtnsControl (strict)"("Disabled"=w821) -> ()  [unwired: 2 in, 2 out]
            n640 = case shown="False" "Optical Switch OPEN" {
              frame False {
                # "Send 2 signals, one for LED indicator, one for switch"
                n641 = Build Array(FALSE, FALSE) -> (w835:bool[])
                n642 = local read "Laser Input Name"() -> (w833:refnum<visa-resource-name>)
                n643 = call "DAQ Assistant3"("data"=w835) -> ()  [unwired: 17 in, 2 out]
                n644 = call "iBs.vi"("Laser On/Off"=FALSE, "VISA resource name"=w833) -> ()
              }
              frame True {
                n645 = Build Array(TRUE, TRUE) -> (w840:bool[])
                n646 = local read "Laser Input Name"() -> (w838:refnum<visa-resource-name>)
                n647 = call "DAQ Assistant4"("data"=w840) -> ()  [unwired: 17 in, 2 out]
                n648 = call "iBs.vi"("Laser On/Off"=TRUE, "VISA resource name"=w838) -> ()
              }
            }
            n649 = Current VI's Menubar() -> (w824:refnum<k9>)
            n650 = case shown="True" "ISS Lasers ON" {
              frame False {
                n651 = Build Array(FALSE) -> (w829:bool[])
                n652 = call "DAQ Assistant5"("data"=w829) -> ()  [unwired: 17 in, 2 out]
              }
              frame True {
                n653 = Build Array(TRUE) -> (w831:bool[])
                n654 = call "DAQ Assistant6"("data"=w831) -> ()  [unwired: 17 in, 2 out]
              }
            }
            n655 = Set Menu Item Info(7:"File", 9:w822, 11:w824) -> (3:w823:refnum<k9>)  [unwired: 4 in, 1 out]
            n656 = Set Menu Item Info(7:"Options", 9:w822, 11:w823) -> ()  [unwired: 4 in, 2 out]
            n657 = Get Date/Time In Seconds() -> (seconds since 1Jan1904=w827:timestamp)
            n658 = Format Date/Time String(seconds (now)=w827) -> (date/time string=w828:string)  [unwired: 2 in]
            n659 = local write "Computer Time"(w828) -> ()
          }
        }
      }
    }
  }
  n660 = local read "Laser Input Name"() -> (w10:refnum<visa-resource-name>)
  n661 = call "iBs.vi"("Laser On/Off"=FALSE, "VISA resource name"=w10) -> ()
  "Trial In Progress" <- FALSE ("Trial In Progress")
  "Acquiring Max" <- FALSE ("Acquiring Max")
